vi "Autonomous Independent.vi"() -> ()   [LabVIEW 2020]
doc: "This VI is called when autonomous begins, and will automatically be terminated when autonomous ends. You can carry out timed or sensor driven robot movement independently without needing to return to the caller."
uses:
  <vilib>/Rock Robotics/WPI/ThirdParty/Phoenix-LabVIEW/Motor Controller/Controls/CTRE_Phoenix_MotorControl_ControlMode.ctl
  <vilib>/Rock Robotics/WPI/Solenoid/WPI_SolenoidSetEnum.vi
  <vilib>/Rock Robotics/WPI/Solenoid/WPI_SolenoidValue.ctl
  <vilib>/Rock Robotics/Network Tables/NT Read Number.vi
  <vilib>/Rock Robotics/Network Tables/NT Read String.vi
  <vilib>/Rock Robotics/Network Tables/NT Write Numeric Array.vi
  AutonBoolean.vi
panel:
  out "Ty 24":dbl
  out "Ty 23":dbl
  out "Ty 22":dbl
  out "Ty 21":dbl
  out "Ty 20":dbl
  out "Ty 19":dbl
  out "Ty 18":dbl
  out "Ty 17":dbl
  out "Orange Limit Pressed 10":bool
  out "Blue Limit Pressed 10":bool
  out "Ty 16":dbl
  out "Orange Limit Pressed 9":bool
  out "Blue Limit Pressed 9":bool
  out "Ty 15":dbl
  out "Intake 5":bool
  out "Elevate 5":bool
  out "Ty 14":dbl
  out "Ty 13":dbl
  out "Ty 12":dbl
  out "Ty 11":dbl
  out "Ty 10":dbl
  out "Ty 9":dbl
  out "Orange Limit Pressed 4":bool
  out "Blue Limit Pressed 4":bool
  out "Ty 4":dbl
  out "Orange Limit Pressed 3":bool
  out "Blue Limit Pressed 3":bool
  out "Ty 3":dbl
  out "Intake 2":bool
  out "Elevate 2":bool
  out "Intake":bool
  out "Elevate":bool
  out "Orange Limit Pressed":bool
  out "Blue Limit Pressed":bool
  out "Ty":dbl
  out "Orange Limit Pressed 2":bool
  out "Blue Limit Pressed 2":bool
  out "Ty 2":dbl
  out "Intake 3":bool
  out "Elevate 3":bool
  out "Orange Limit Pressed 5":bool
  out "Blue Limit Pressed 5":bool
  out "Ty 5":dbl
  out "Orange Limit Pressed 6":bool
  out "Blue Limit Pressed 6":bool
  out "Ty 6":dbl
  out "Intake 4":bool
  out "Elevate 4":bool
  out "Orange Limit Pressed 7":bool
  out "Blue Limit Pressed 7":bool
  out "Ty 7":dbl
  out "Orange Limit Pressed 8":bool
  out "Blue Limit Pressed 8":bool
  out "Ty 8":dbl
  # "Be sure to right-click and choose Data Operations>>Make Current Value default if you want to save the array values with the VI"
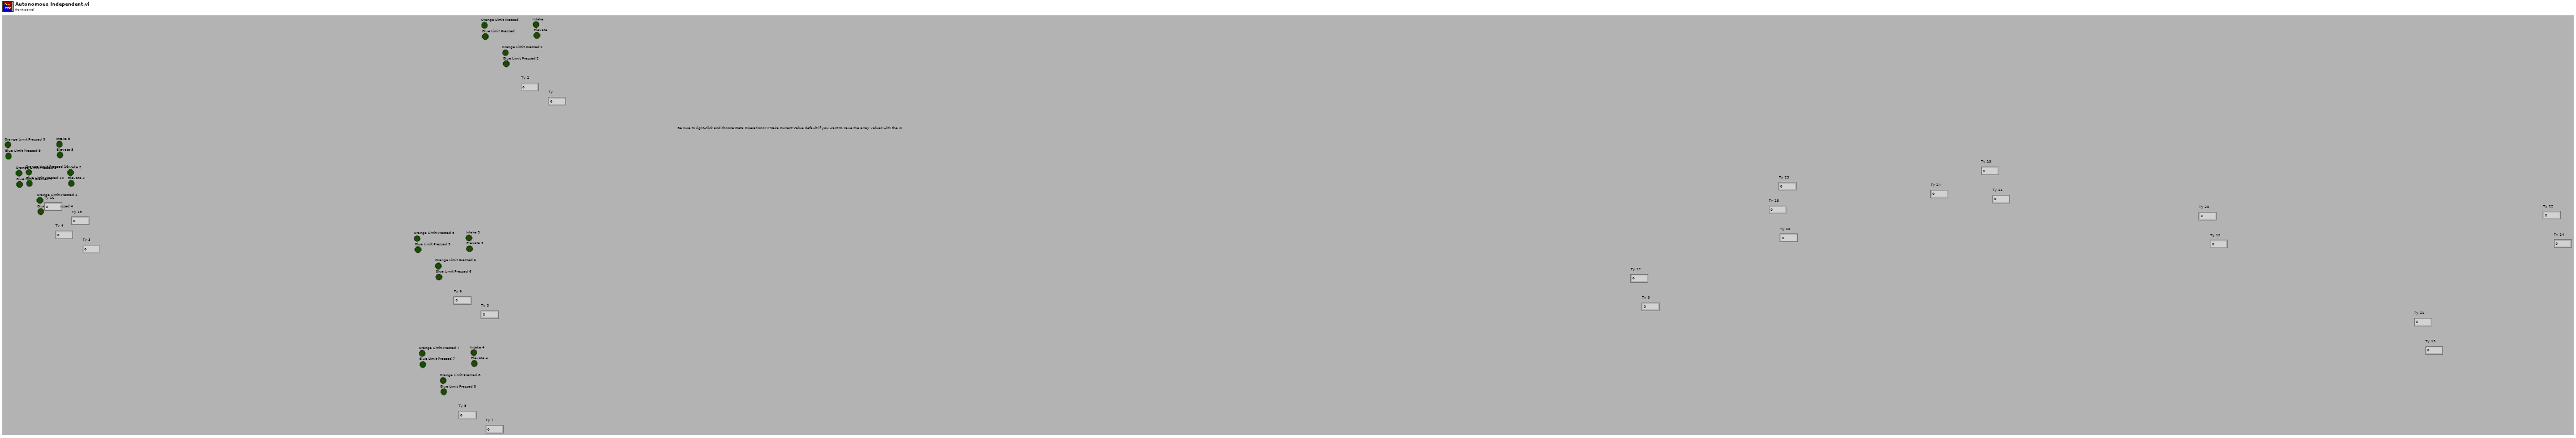
[diagram p1: front panel]
types:
  T1 = typedef "WPI_JoystickDevRef.ctl" = cluster{"Device":T2}
  T2 = typedef "WPI_JoystickDeviceEnum.ctl" = enum16{"USB 0", "USB 1", "USB 2", "USB 3", "USB 4", "USB 5"}
  T3 = typedef "WPI_SolenoidValue.ctl" = enum16{"Off", "On", "Forward", "Reverse"}
  T4 = typedef "WPI_SwitchDevRef.ctl" = cluster{"DevStatus":errorcluster, "DIO Channel":T5, "CntIndex":T6, "Normally Closed":bool}
  T5 = typedef "FPGA_DIOChannel.ctl" = enum8{"DIO 0", "DIO 1", "DIO 2", "DIO 3", "DIO 4", "DIO 5", "DIO 6", "DIO 7", "DIO 8", "DIO 9", "DIO MXP 0", "DIO MXP 1", "DIO MXP 2", "DIO MXP 3", "DIO MXP 4", "DIO MXP 5", "DIO MXP 6", "DIO MXP 7", "DIO MXP 8", "DIO MXP 9", "DIO MXP 10", "DIO MXP 11", "DIO MXP 12", "DIO MXP 13", "DIO MXP 14", "DIO MXP 15", "SPI Port CS1", "SPI Port CS2", "SPI Port CS3", "SPI Port MISO", "SPI Port MOSI", "Invalid"}
  T6 = typedef "FPGA_CounterCtrSystemIndex.ctl" = enum8{"Ctr 0", "Ctr 1", "Ctr 2", "Ctr 3", "Ctr 4", "Ctr 5", "Ctr 6", "Ctr 7", "Invalid"}
  T7 = typedef "WPI_SolenoidDevRef.ctl" = cluster{"DevStatus":errorcluster, "Pneumatics Control Module":u8, "Forward Solenoid Channel":T8, "Reverse Solenoid Channel":T8}
  T8 = typedef "WPI_SolenoidChannel.ctl" = enum8{"Solenoid 0", "Solenoid 1", "Solenoid 2", "Solenoid 3", "Solenoid 4", "Solenoid 5", "Solenoid 6", "Solenoid 7", "Solenoid 8", "Solenoid 9", "Solenoid 10", "Solenoid 11", "Solenoid 12", "Solenoid 13", "Solenoid 14", "Solenoid 15", "Invalid"}
  T9 = typedef "WPI_MotorControlDeviceRef.ctl" = cluster{"DeviceStatus":errorcluster, "Type":T10, "PWM":cluster{"PWM Channel":T11, "DeadBand":T12}, "CAN":cluster{"Device Number":u8, "SetOutput VI Ref":variant, "GetOutput VI Ref":variant, "Enable VI Ref":variant, "Disable VI Ref":variant, "Data":variant}, "Invert":bool, "DIO PWM":cluster{"PWM \"Enable\" Channel":T11, "DIOChannel":T5, "PWM Rate":dbl}}
  T10 = typedef "WPI_MotorControlType.ctl" = enum16{"PWM", "CAN", "DIO PWM"}
  T11 = typedef "FPGA_DIOPWMChannel.ctl" = enum8{"PWM 0", "PWM 1", "PWM 2", "PWM 3", "PWM 4", "PWM 5", "PWM 6", "PWM 7", "PWM 8", "PWM 9", "PWM MXP 0", "PWM MXP 1", "PWM MXP 2", "PWM MXP 3", "PWM MXP 4", "PWM MXP 5", "PWM MXP 6", "PWM MXP 7", "PWM MXP 8", "PWM MXP 9", "Invalid"}
  T12 = typedef "WPI_PWMDeadband.ctl" = cluster{"Name":string, "maxPositivePwm":i32, "minPositivePwm":i32, "centerPwm":i32, "maxNegativePwm":i32, "minNegativePwm":i32, "angularRange":u16}
  T13 = typedef "CTRE_Phoenix_MotorControl_ControlMode.ctl" = u16
  T14 = typedef "Trajectory Data.ctl" = cluster{"Segment Name":string, "Type":T15, "Traj Pos Points":cluster{"x":dbl, "y":dbl, "th":dbl}[], "Traj Vel Points":cluster{"V":dbl, "Omega":dbl, "V vector":cluster{"y":dbl, "x":dbl}}[], "Accel Index":i32, "Decel Index":i32}[]
  T15 = typedef "Segment Type.ctl" = enum16{"Accel Straight", "Const Straight", "Blend", "Circle", "Bezier"}
  T16 = typedef "Overrides.ctl" = cluster{"Count":string, "Angular Override":dbl, "Enabled?":bool, "Velocity Override":dbl, "Angle Override":dbl}[]
  T17 = typedef "Angluar Limits.ctl" = cluster{"Velocity (deg/s)":dbl, "Accel (deg/s^2)":dbl, "Jerk (deg/s^3)":dbl}
  T18 = cluster{"Sample Period (s)":dbl, cluster{"Velocity (fps)":dbl, "Accel (fps^2)":dbl, "Jerk (fps^3)":dbl, "StoopidFast (fps)":dbl}, "Conditions":cluster{"vInitial (fps)":dbl, "vFinal (fps)":dbl}, "Overrides":T16, "Angular Limits":T17}
  T19 = cluster{"Velocity (fps)":dbl, "Accel (fps^2)":dbl, "Jerk (fps^3)":dbl, "StoopidFast (fps)":dbl}
  T20 = cluster{"V":dbl, "Omega":dbl, "V vector":cluster{"y":dbl, "x":dbl}}[]
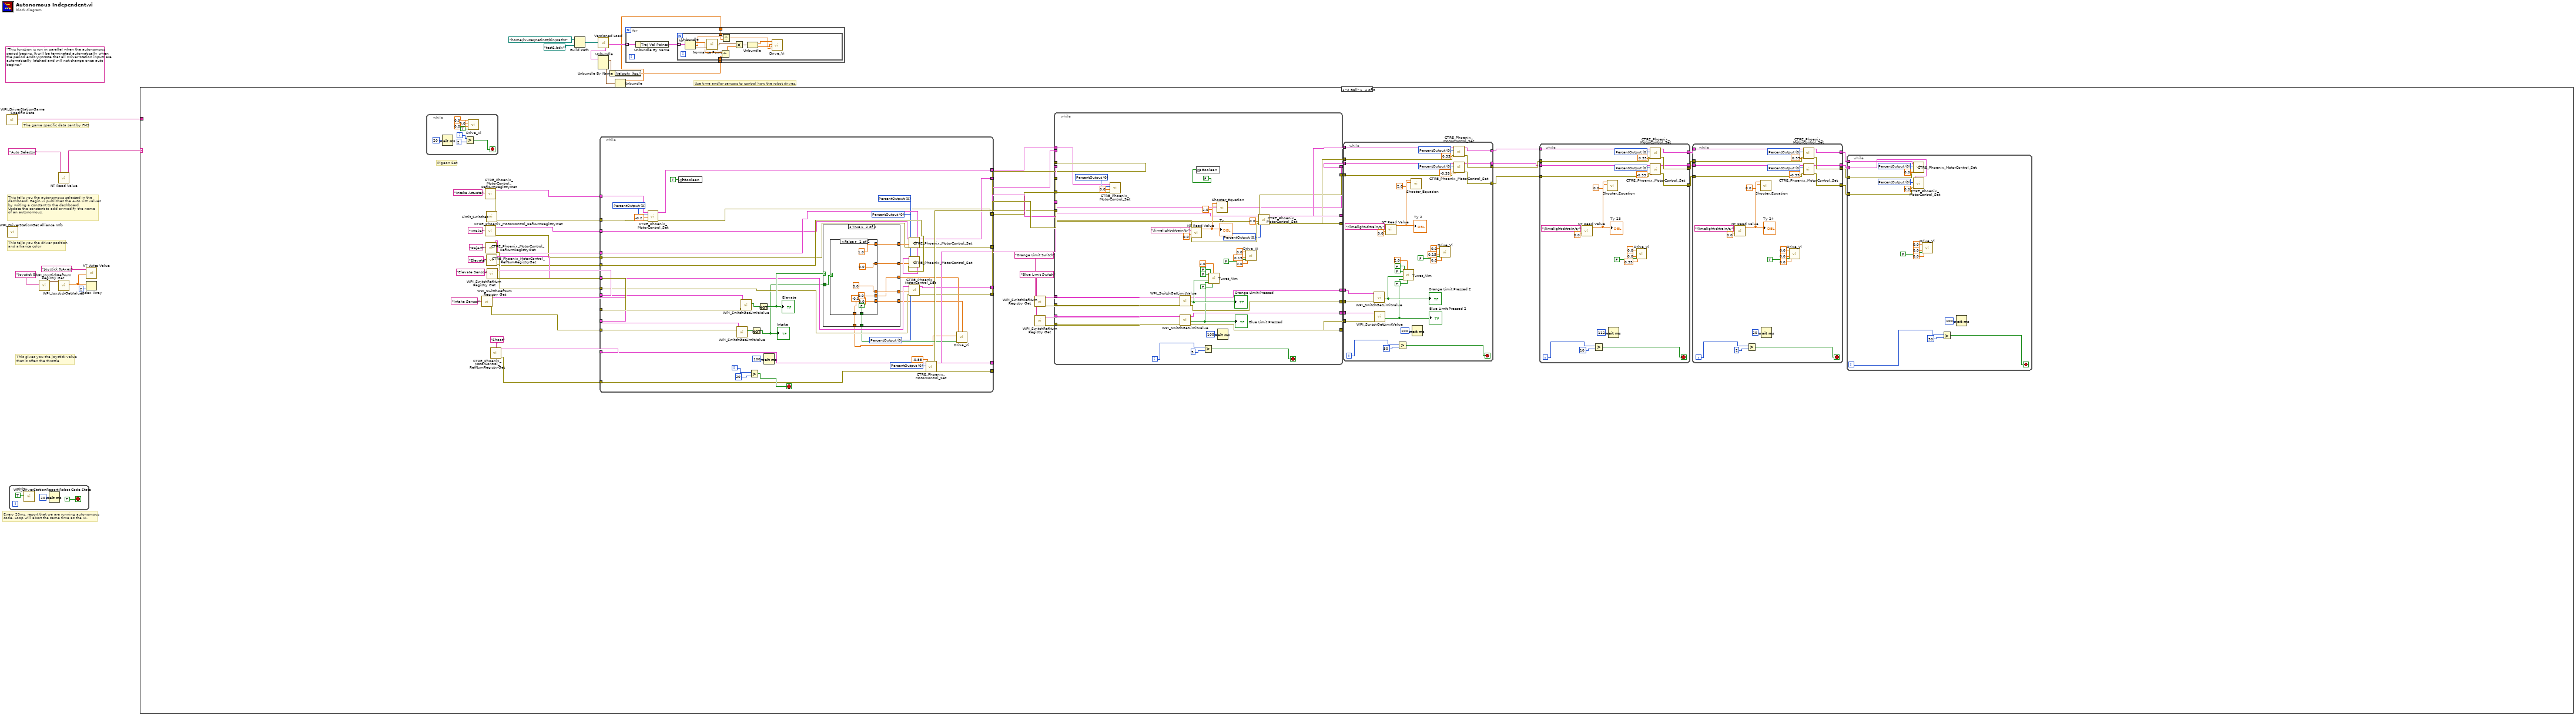
[diagram p0: block diagram]
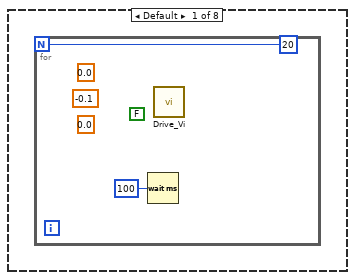
[diagram p2: hidden frame]
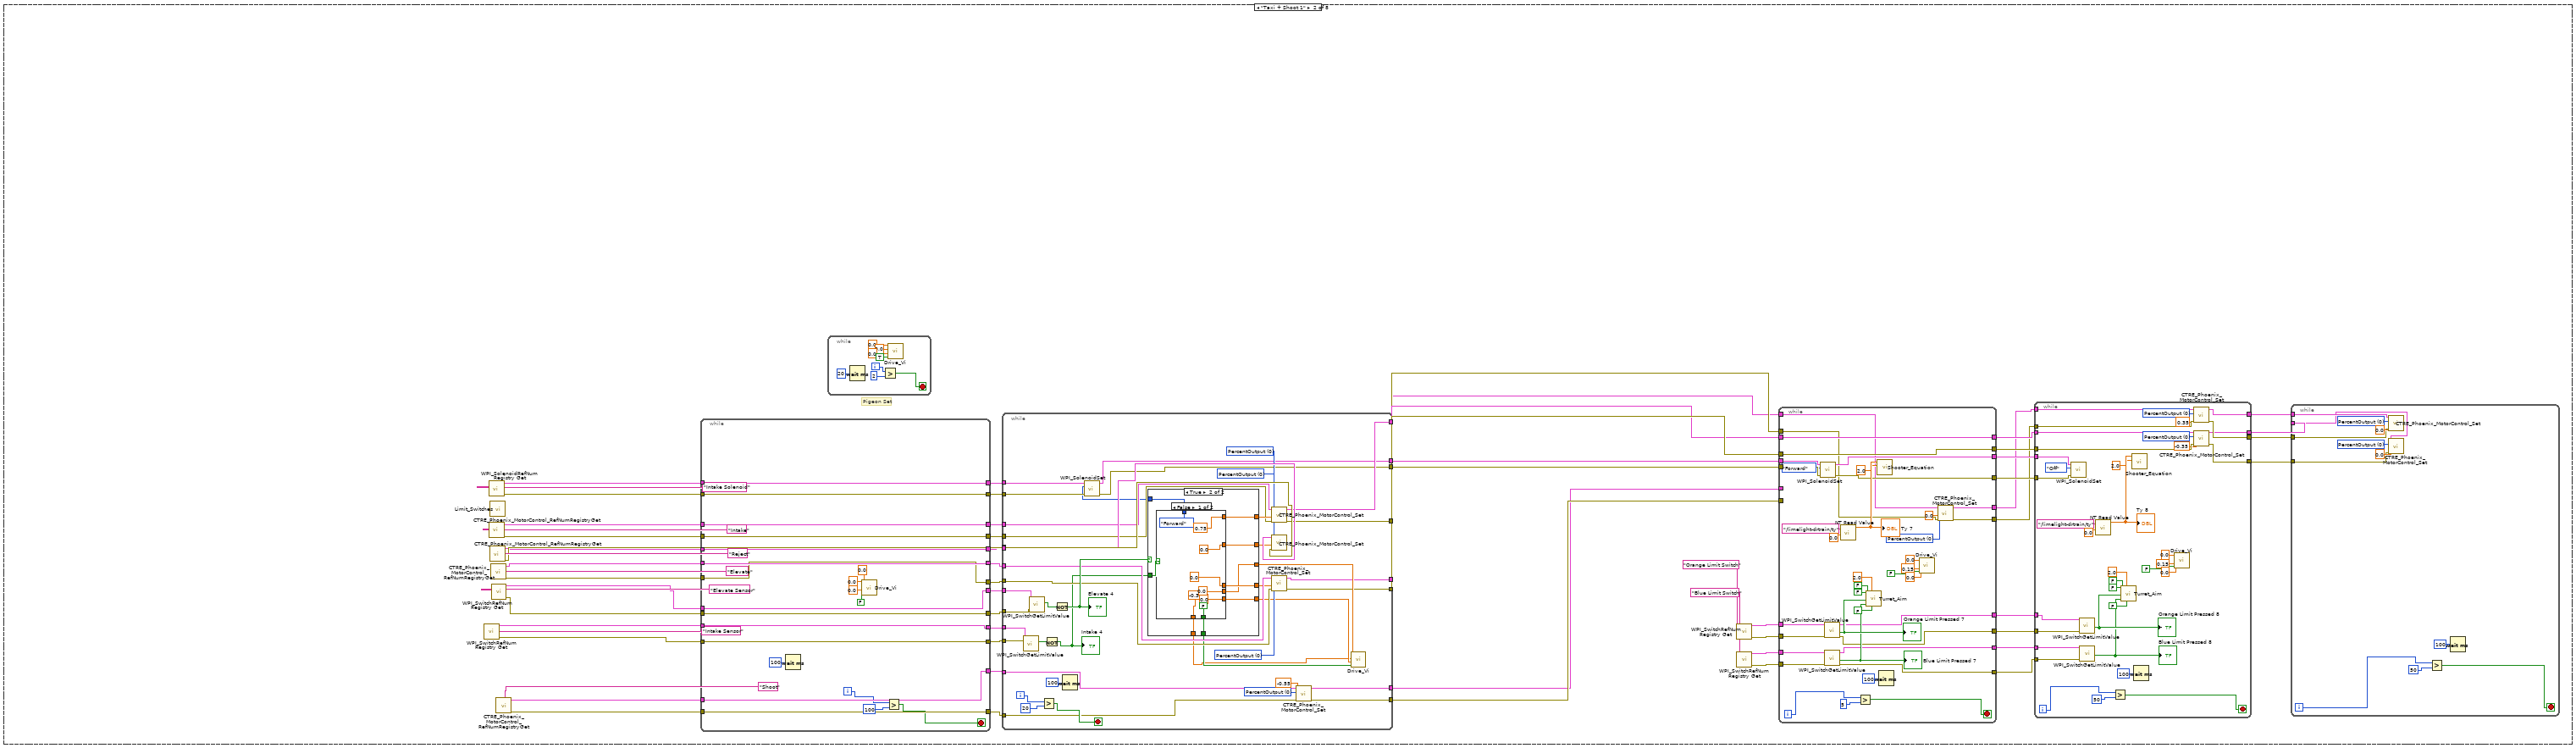
[diagram p3: hidden frame]
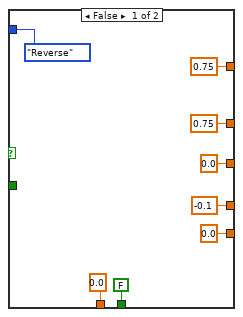
[diagram p4: hidden frame]
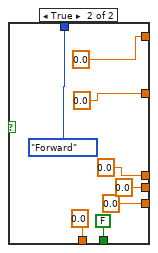
[diagram p5: hidden frame]
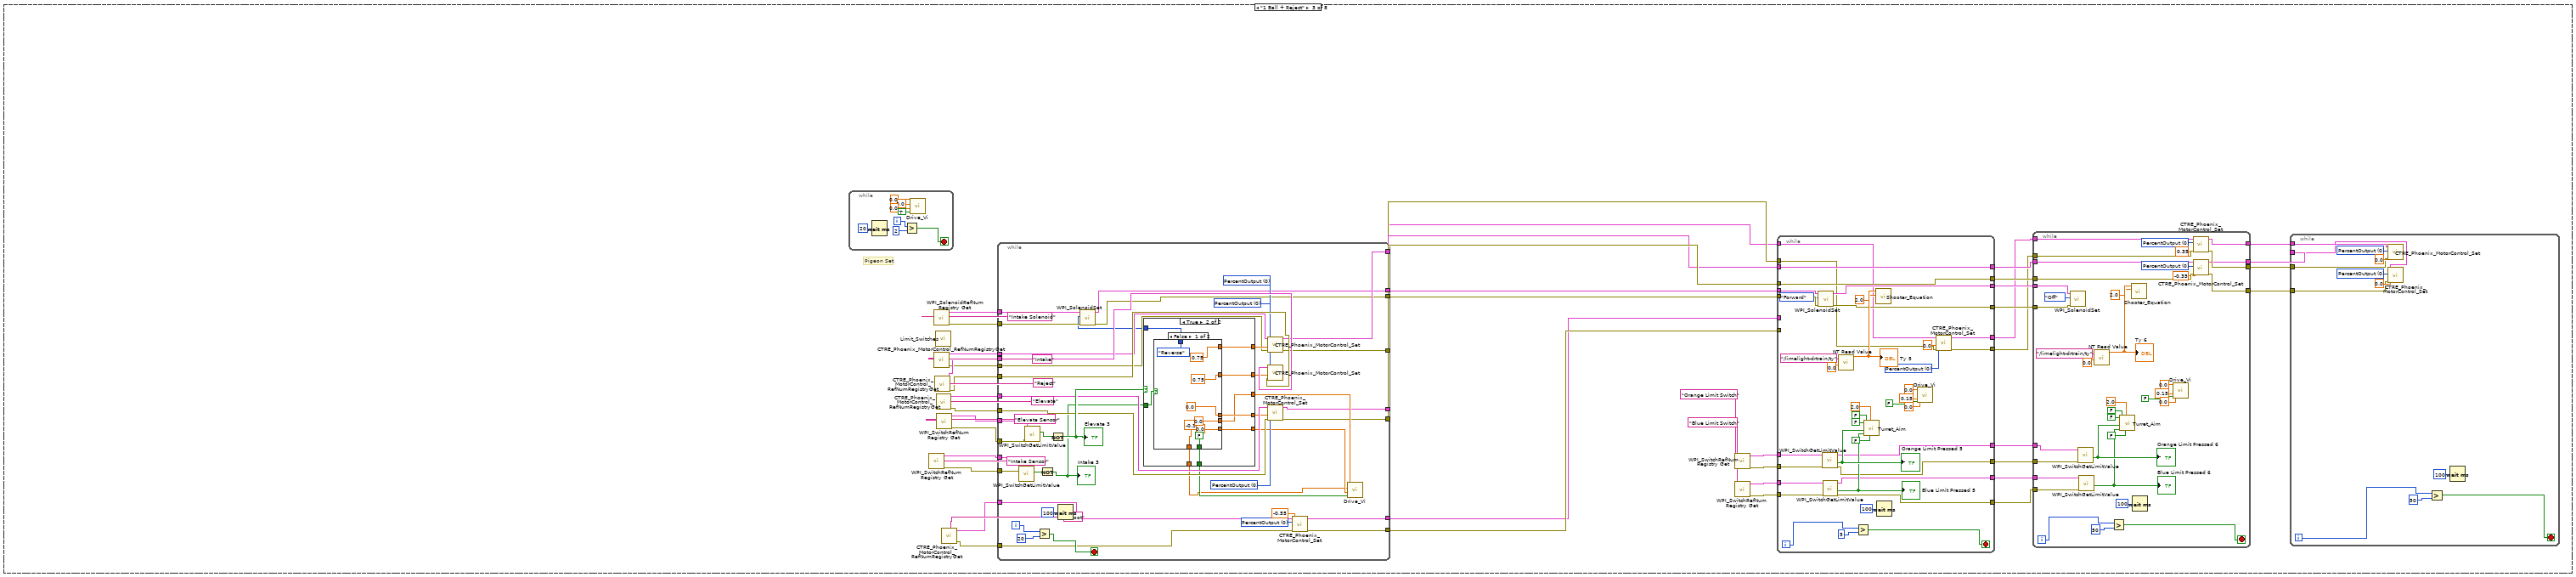
[diagram p6: hidden frame]
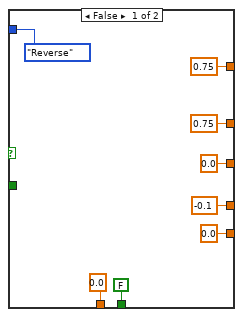
[diagram p7: hidden frame]
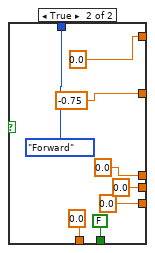
[diagram p8: hidden frame]
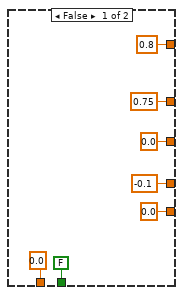
[diagram p9: hidden frame]
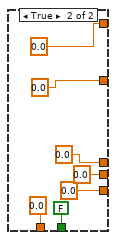
[diagram p10: hidden frame]
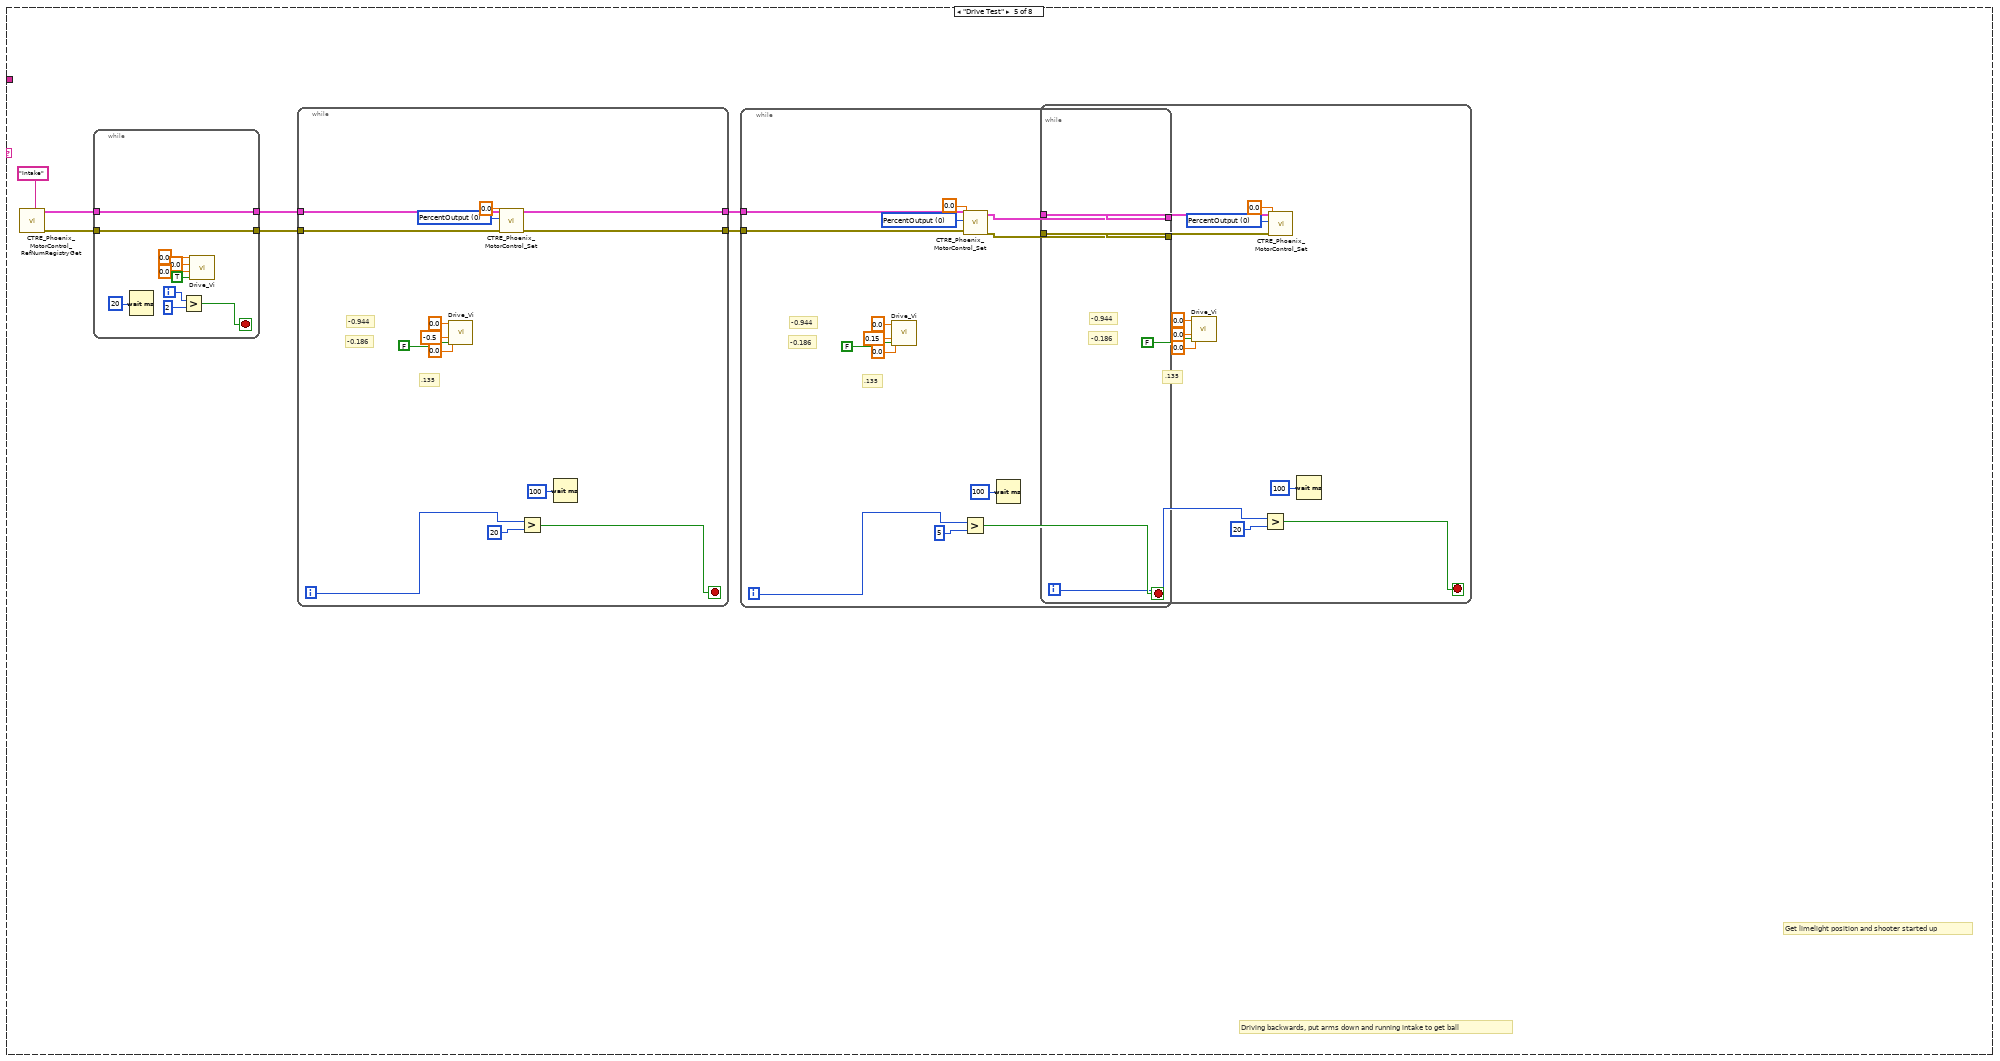
[diagram p11: hidden frame]
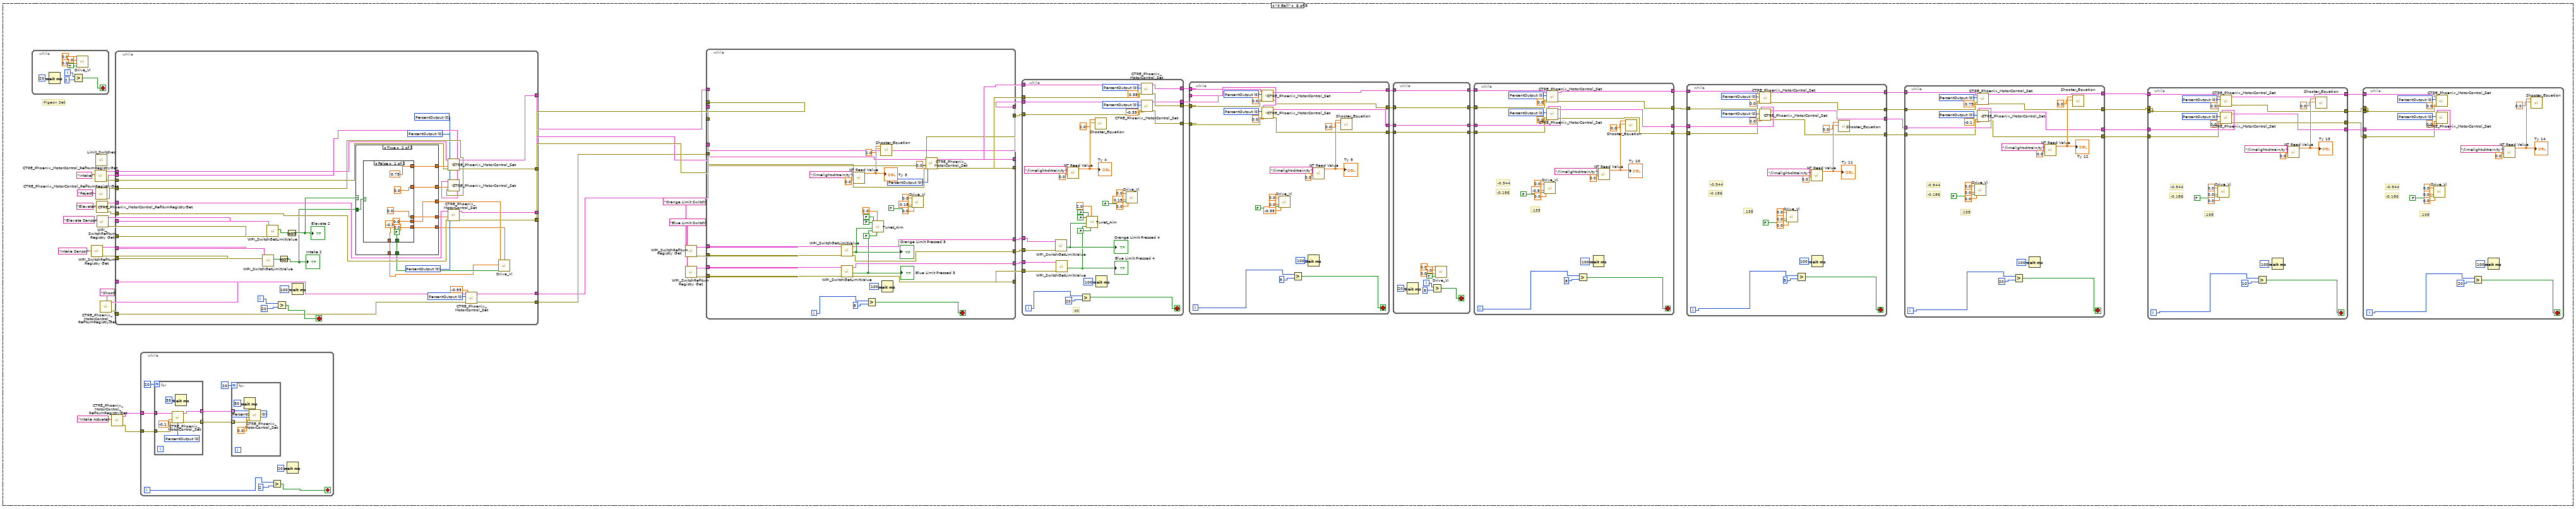
[diagram p12: hidden frame]
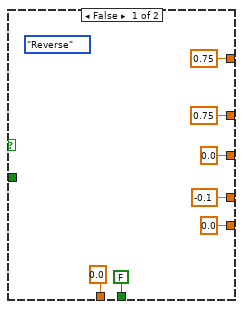
[diagram p13: hidden frame]
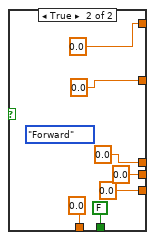
[diagram p14: hidden frame]
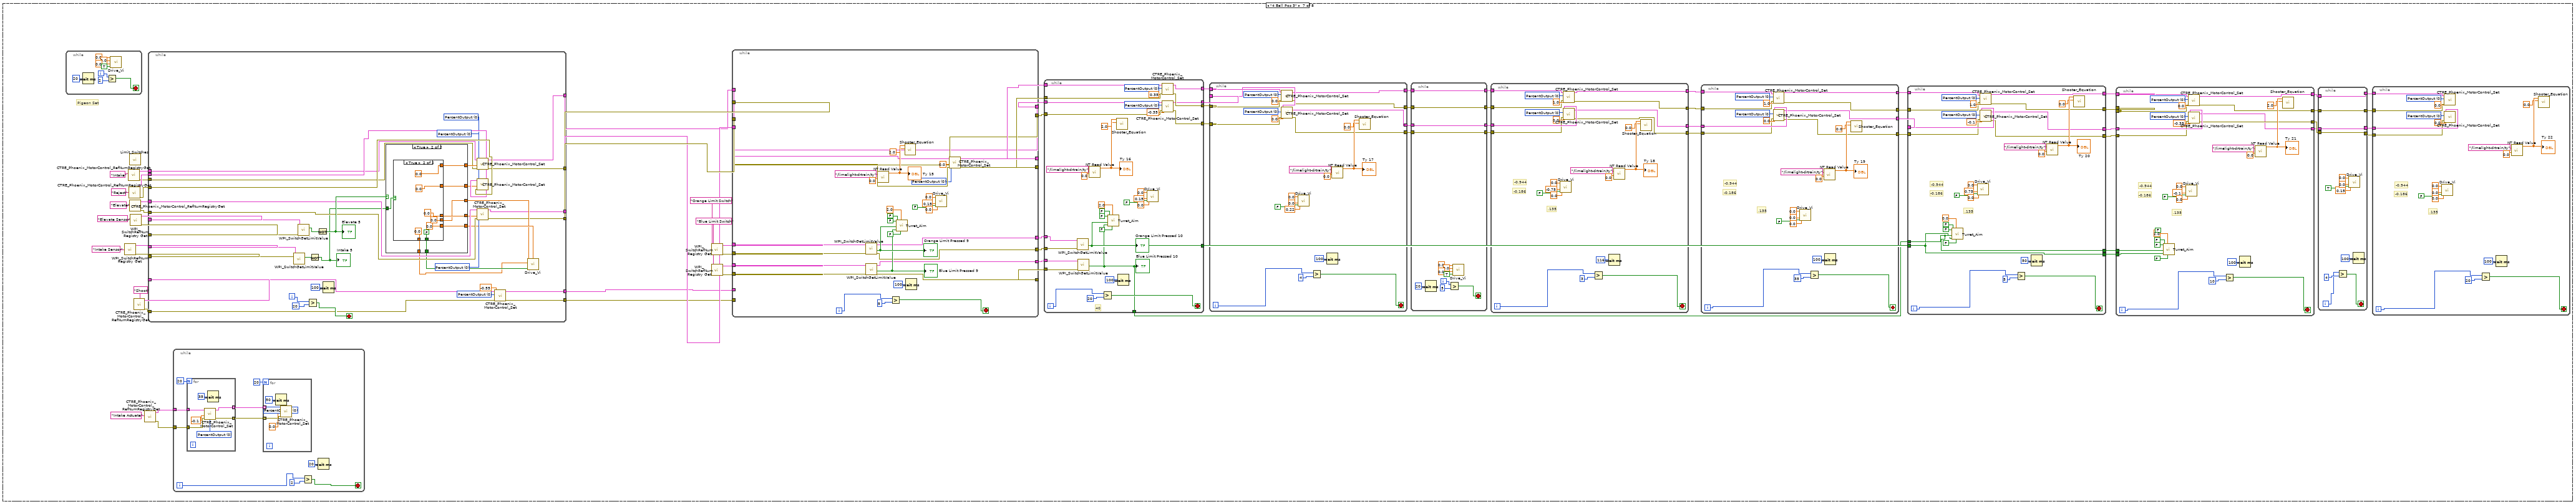
[diagram p15: hidden frame]
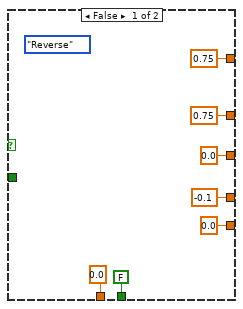
[diagram p16: hidden frame]
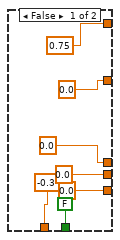
[diagram p17: hidden frame]
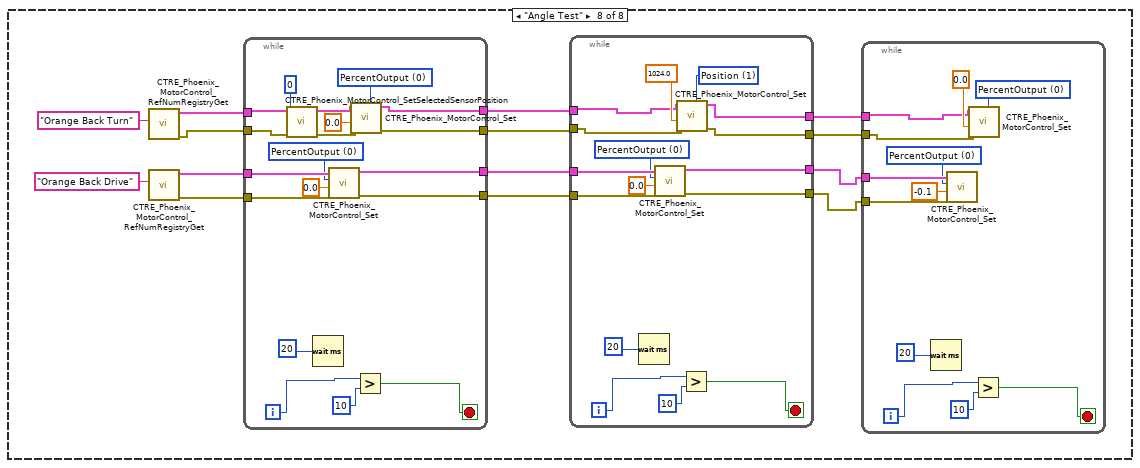
[diagram p18: hidden frame]
diagram:
  (unwired) "This function is run in parallel when the autonomous period begins. It will be terminated automatically when the period ends.\n\nNote that all Driver Station inputs are automatically latched and will not change once auto begins."
  # "The game specific data sent by FMS"
  # "This tells you the autonomous selected in the \ndashboard. Begin.vi publishes the Auto List values\nby writing a constant to the dashboard.\nUpdate the constant to add or modify the name\nof an autonomous."
  # "Every 20ms, report that we are running autonomous\ncode. Loop will abort the same time as the VI."
  # "This gives you the joystick value\nthat is often the throttle"
  # "Use time and/or sensors to control how the robot drives."
  # "This tells you the driver position\nand alliance color"
  n1 = call <vilib>:"WPI_DriverStationGame Specific Data.vi"() -> ("Game Specific Data"=w10:string)  [unwired: 11 in]
  n2 = call <vilib>:"WPI_DriverStationGet Alliance Info.vi"() -> ()  [unwired: 12 out]
  n3 = while {
    stop <- FALSE stop-if-true
    n4 = call <vilib>:"WPI_DriverStationReport Robot Code State.vi"("Autonomous"=TRUE) -> ()  [unwired: 10 in, 1 out]
    n5 = Wait (ms)(milliseconds to wait=u32 20) -> ()  [unwired: 1 out]
  }
  n6 = call <vilib>:"WPI_JoystickRefNum Registry Get.vi"("refnum name"="Joystick 0") -> ("JoystickDevRef"=w16:T1)  [unwired: 1 in, 9 out]
  n7 = call <vilib>:"WPI_JoystickGetValues.vi"("JoystickDevRef"=w16) -> ("Axes"=w12:dbl[])  [unwired: 6 in, 4 out]
  n8 = call-poly <vilib>:"NT Read Value.vi"("Name"="Auto Selector") -> ("String"=w13:string)  [unwired: 9 in, 1 out]
  n9 = call-poly <vilib>:"NT Write Value.vi"("Numeric Array"=w12, "Name"="Joystick 0/Axes") -> ()  [unwired: 9 in, 1 out]
  n10 = Index Array(array=w12, index=2) -> ()  [unwired: 1 out]
  n11 = case shown="\"2 Ball\"" w13 {
    tunnel: w10 -> [_ _ _ _ _ _ _ _]
    frame Default {
      n12 = for {
        N: 20 -> [_]
        (unwired) FALSE ("Middle Thumb")
        (unwired) 0.0 ("Z")
        (unwired) -0.1 ("Y")
        (unwired) 0.0 ("X")
        n13 = Wait (ms)(milliseconds to wait=u32 100) -> ()  [unwired: 1 out]
        n14 = call "Drive_Vi.vi"() -> ()  [unwired: 12 in]
      }
    }
    frame "Taxi + Shoot 1" {
      # "Pigeon Set"
      n15 = call <vilib>:"WPI_SwitchRefNum Registry Get.vi"("refnum name"="Intake Sensor") -> ("error out"=w27:errorcluster, "SwitchDevRef"=w29:T4)  [unwired: 9 in]
      n16 = call <vilib>:"WPI_SolenoidRefNum Registry Get.vi"("refnum name"="Intake Solenoid") -> ("error out"=w46:errorcluster, "SolenoidDevRef"=w48:T7)  [unwired: 9 in]
      n17 = call <vilib>:"CTRE_Phoenix_MotorControl_RefNumRegistryGet.vi"("refnum name"="Intake") -> ("error out"=w41:errorcluster, "PhoenixMotorControlDevRef"=w43:T9)  [unwired: 9 in]
      n18 = call <vilib>:"CTRE_Phoenix_MotorControl_RefNumRegistryGet.vi"("refnum name"="Reject") -> ("error out"=w77:errorcluster, "PhoenixMotorControlDevRef"=w39:T9)  [unwired: 9 in]
      n19 = call "Limit_Switches.vi"() -> ()  [unwired: 10 in, 2 out]
      n20 = call <vilib>:"CTRE_Phoenix_MotorControl_RefNumRegistryGet.vi"("refnum name"="Elevate") -> ("error out"=w35:errorcluster, "PhoenixMotorControlDevRef"=w37:T9)  [unwired: 9 in]
      n21 = call <vilib>:"WPI_SwitchRefNum Registry Get.vi"("refnum name"="Elevate Sensor") -> ("error out"=w31:errorcluster, "SwitchDevRef"=w33:T4)  [unwired: 9 in]
      n22 = call <vilib>:"CTRE_Phoenix_MotorControl_RefNumRegistryGet.vi"("refnum name"="Shoot") -> ("error out"=w23:errorcluster, "PhoenixMotorControlDevRef"=w26:T9)  [unwired: 9 in]
      n23 = while {
        tunnel: [w101] -> w47
        tunnel: w48 -> [w101]
        tunnel: [w100] -> w45
        tunnel: w46 -> [w100]
        tunnel: [w99] -> w44
        tunnel: w43 -> [w99]
        tunnel: [w98] -> w42
        tunnel: w41 -> [w98]
        tunnel: [w97] -> w40
        tunnel: w39 -> [w97]
        tunnel: [w96] -> w38
        tunnel: w37 -> [w96]
        tunnel: [w95] -> w36
        tunnel: w35 -> [w95]
        tunnel: [w94] -> w34
        tunnel: w33 -> [w94]
        tunnel: [w93] -> w32
        tunnel: w31 -> [w93]
        tunnel: [w92] -> w30
        tunnel: w29 -> [w92]
        tunnel: [w91] -> w28
        tunnel: w27 -> [w91]
        tunnel: [w90] -> w25
        tunnel: w26 -> [w90]
        tunnel: [w89] -> w24
        tunnel: w23 -> [w89]
        i -> [w85]
        stop <- w87 stop-if-true
        n24 = Wait (ms)(milliseconds to wait=u32 100) -> ()  [unwired: 1 out]
        n25 = call "Drive_Vi.vi"("Middle Thumb"=FALSE, "Z"=0.0, "Y"=0.0, "X"=0.0) -> ()  [unwired: 8 in]
        n26 = Greater?(x=w85, y=100) -> (0:w87:bool)
      }
      n27 = while {
        i -> [w275]
        stop <- w276 stop-if-true
        n28 = Wait (ms)(milliseconds to wait=u32 20) -> ()  [unwired: 1 out]
        n29 = Greater?(x=w275, y=2) -> (0:w276:bool)
        n30 = call "Drive_Vi.vi"("Middle Thumb"=TRUE, "Z"=0.0, "Y"=0.0, "X"=0.0) -> ()  [unwired: 8 in]
      }
      n31 = while {
        tunnel: w32 -> [w230]
        tunnel: w34 -> [w229]
        tunnel: w28 -> [w228]
        tunnel: w30 -> [w227]
        tunnel: w45 -> [w226]
        tunnel: w47 -> [w225]
        tunnel: w36 -> [w222]
        tunnel: w38 -> [w221]
        tunnel: w77 -> [w220]
        tunnel: w40 -> [w219]
        tunnel: w42 -> [w218]
        tunnel: w44 -> [w217]
        tunnel: [w205] -> w70
        tunnel: [w204] -> w69
        tunnel: [w203] -> w68
        tunnel: [w202] -> w67
        tunnel: w24 -> [w201]
        tunnel: w25 -> [w200]
        tunnel: [w197] -> w66
        tunnel: [w196] -> w65
        tunnel: [w195] -> w58
        tunnel: [w194] -> w57
        i -> [w233]
        stop <- w234 stop-if-true
        w199 = T13 0 items=["PercentOutput"=0, "Position"=1, "Velocity"=2, "Current"=3, "Follower"=5, "MotionProfile"=6, "MotionMagic"=7, "MotionProfileArc"=10, "Disabled"=15] ("Control Mode")
        w211 = T13 0 items=["PercentOutput"=0, "Position"=1, "Velocity"=2, "Current"=3, "Follower"=5, "MotionProfile"=6, "MotionMagic"=7, "MotionProfileArc"=10, "Disabled"=15] ("Control Mode")
        w212 = T13 0 items=["PercentOutput"=0, "Position"=1, "Velocity"=2, "Current"=3, "Follower"=5, "MotionProfile"=6, "MotionMagic"=7, "MotionProfileArc"=10, "Disabled"=15] ("Control Mode")
        w213 = T13 0 items=["PercentOutput"=0, "Position"=1, "Velocity"=2, "Current"=3, "Follower"=5, "MotionProfile"=6, "MotionMagic"=7, "MotionProfileArc"=10, "Disabled"=15] ("Control Mode")
        n32 = call <vilib>:"WPI_SwitchGetLimitValue.vi"("error in (no error)"=w228, "SwitchDevRef"=w227) -> ("Switch Pressed"=w231:bool)  [unwired: 7 in, 2 out]
        n33 = call <vilib>:"WPI_SwitchGetLimitValue.vi"("error in (no error)"=w230, "SwitchDevRef"=w229) -> ("Switch Pressed"=w232:bool)  [unwired: 7 in, 2 out]
        n34 = Greater?(x=w233, y=20) -> (0:w234:bool)
        n35 = Not(x=w231) -> (.not. x?=w216:bool)
        "Intake 4" <- w216
        n36 = Not(x=w232) -> (.not. x?=w224:bool)
        "Elevate 4" <- w224
        n37 = Wait (ms)(milliseconds to wait=u32 100) -> ()  [unwired: 1 out]
        n38 = case shown="True" w224 {
          tunnel: [0.75 ("Output") w253] -> w223
          tunnel: w216 -> [_ w250]
          tunnel: [0.75 ("Output") w252] -> w215
          tunnel: [-0.1 ("Output") w251] -> w214
          tunnel: [FALSE ("Middle Thumb") w249] -> w210
          tunnel: [0.0 ("Z") w248] -> w209
          tunnel: [0.0 ("Y") w247] -> w208
          tunnel: [0.0 ("X") w246] -> w207
          tunnel: [WPI_SolenoidValue."Reverse" ("Value") w245] -> w206
          frame False {
          }
          frame True {
            n39 = case shown="False" w250 {
              tunnel: [0.75 ("Output") 0.0 ("Output")] -> w253
              tunnel: [0.0 ("Output") 0.0 ("Output")] -> w252
              tunnel: [0.0 ("Output") 0.0 ("Output")] -> w251
              tunnel: [FALSE ("Middle Thumb") FALSE ("Middle Thumb")] -> w249
              tunnel: [0.0 ("Z") 0.0 ("Z")] -> w248
              tunnel: [-0.3 ("Y") 0.0 ("Y")] -> w247
              tunnel: [0.0 ("X") 0.0 ("X")] -> w246
              tunnel: [WPI_SolenoidValue."Forward" ("Value") WPI_SolenoidValue."Forward" ("Value")] -> w245
              frame False {
              }
              frame True {
              }
            }
          }
        }
        n40 = call-poly <vilib>:"WPI_SolenoidSet.vi"("error in (no error)"=w226, "Value"=w206, "SolenoidDevRef"=w225) -> ("error out"=w194:errorcluster, "SolenoidDevRef"=w195:T7)  [unwired: 7 in]
        n41 = call <vilib>:"CTRE_Phoenix_MotorControl_Set.vi"("error in (no error)"=w218, "Output"=w223, "Control Mode"=w211, "PhoenixMotorControlDevRef"=w217) -> ("error out"=w203:errorcluster, "PhoenixMotorControlDevRef"=w202:T9)  [unwired: 6 in]
        n42 = call <vilib>:"CTRE_Phoenix_MotorControl_Set.vi"("error in (no error)"=w220, "Output"=w215, "Control Mode"=w212, "PhoenixMotorControlDevRef"=w219) -> ()  [unwired: 6 in, 2 out]
        n43 = call <vilib>:"CTRE_Phoenix_MotorControl_Set.vi"("error in (no error)"=w222, "Output"=w214, "Control Mode"=w213, "PhoenixMotorControlDevRef"=w221) -> ("error out"=w205:errorcluster, "PhoenixMotorControlDevRef"=w204:T9)  [unwired: 6 in]
        n44 = call <vilib>:"CTRE_Phoenix_MotorControl_Set.vi"("error in (no error)"=w201, "Output"=-0.55, "Control Mode"=w199, "PhoenixMotorControlDevRef"=w200) -> ("error out"=w197:errorcluster, "PhoenixMotorControlDevRef"=w196:T9)  [unwired: 6 in]
        n45 = call "Drive_Vi.vi"("Middle Thumb"=w210, "Z"=w209, "Y"=w208, "X"=w207) -> ()  [unwired: 8 in]
      }
      n46 = call <vilib>:"WPI_SwitchRefNum Registry Get.vi"("refnum name"="Orange Limit Switch") -> ("error out"=w72:errorcluster, "SwitchDevRef"=w71:T4)  [unwired: 9 in]
      n47 = call <vilib>:"WPI_SwitchRefNum Registry Get.vi"("refnum name"="Blue Limit Switch") -> ("error out"=w74:errorcluster, "SwitchDevRef"=w73:T4)  [unwired: 9 in]
      n48 = while {
        tunnel: w66 -> [_]
        tunnel: w65 -> [_]
        tunnel: w74 -> [w191]
        tunnel: w73 -> [w190]
        tunnel: w72 -> [w189]
        tunnel: w71 -> [w188]
        tunnel: w70 -> [w167]
        tunnel: w69 -> [w166]
        tunnel: w68 -> [w157]
        tunnel: w67 -> [w158]
        tunnel: [w171] -> w64
        tunnel: [w170] -> w63
        tunnel: [w169] -> w62
        tunnel: [w168] -> w61
        tunnel: [w167] -> w60
        tunnel: [w166] -> w59
        tunnel: w58 -> [w165]
        tunnel: w57 -> [w164]
        tunnel: [w162] -> w56
        tunnel: [w161] -> w55
        tunnel: [w160] -> w54
        tunnel: [w159] -> w53
        i -> [w177]
        stop <- w176 stop-if-true
        w156 = T13 0 items=["PercentOutput"=0, "Position"=1, "Velocity"=2, "Current"=3, "Follower"=5, "MotionProfile"=6, "MotionMagic"=7, "MotionProfileArc"=10, "Disabled"=15] ("Control Mode")
        n49 = call-poly <vilib>:"WPI_SolenoidSet.vi"("error in (no error)"=w164, "Value"=WPI_SolenoidValue."Forward", "SolenoidDevRef"=w165) -> ("error out"=w161:errorcluster, "SolenoidDevRef"=w162:T7)  [unwired: 7 in]
        n50 = call <vilib>:"WPI_SwitchGetLimitValue.vi"("error in (no error)"=w189, "SwitchDevRef"=w188) -> ("error out"=w168:errorcluster, "Switch Pressed"=w187:bool, "SwitchDevRef"=w169:T4)  [unwired: 7 in]
        "Orange Limit Pressed 7" <- w187
        n51 = call <vilib>:"WPI_SwitchGetLimitValue.vi"("error in (no error)"=w191, "SwitchDevRef"=w190) -> ("error out"=w170:errorcluster, "Switch Pressed"=w186:bool, "SwitchDevRef"=w171:T4)  [unwired: 7 in]
        "Blue Limit Pressed 7" <- w186
        n52 = call-poly <vilib>:"NT Read Value.vi"("Default Value"=0.0, "Name"="/limelight-drtrain/ty") -> ("Numeric"=w181:dbl)  [unwired: 8 in, 1 out]
        "Ty 7" <- w181
        n53 = Greater?(x=w177, y=5) -> (0:w176:bool)
        n54 = call "Turret_Aim.vi"("View Button"=FALSE ("Driver Right Thumb"), "Left Trigger"=2.0, "Orange Limit Pressed"=w186, "Blue Limit Pressed"=w187, "Right Bumper"=FALSE, "Left Bumper"=FALSE) -> ()  [unwired: 6 in]
        n55 = call "Shooter_Equation.vi"("Right Trigger"=2.0, "Ty"=w181) -> ()  [unwired: 10 in]
        n56 = Wait (ms)(milliseconds to wait=u32 100) -> ()  [unwired: 1 out]
        n57 = call "Drive_Vi.vi"("Middle Thumb"=FALSE, "Z"=0.0, "Y"=0.15, "X"=0.0) -> ()  [unwired: 8 in]
        n58 = call <vilib>:"CTRE_Phoenix_MotorControl_Set.vi"("error in (no error)"=w157, "Output"=0.0, "Control Mode"=w156, "PhoenixMotorControlDevRef"=w158) -> ("error out"=w159:errorcluster, "PhoenixMotorControlDevRef"=w160:T9)  [unwired: 6 in]
      }
      n59 = while {
        tunnel: w63 -> [w152]
        tunnel: w64 -> [w151]
        tunnel: w61 -> [w150]
        tunnel: w60 -> [w137]
        tunnel: w59 -> [w136]
        tunnel: w53 -> [w135]
        tunnel: w54 -> [w134]
        tunnel: w62 -> [w125]
        tunnel: w56 -> [w124]
        tunnel: w55 -> [w123]
        tunnel: [w121] -> w52
        tunnel: [w120] -> w51
        tunnel: [w119] -> w50
        tunnel: [w118] -> w49
        i -> [w139]
        stop <- w138 stop-if-true
        w132 = T13 0 items=["PercentOutput"=0, "Position"=1, "Velocity"=2, "Current"=3, "Follower"=5, "MotionProfile"=6, "MotionMagic"=7, "MotionProfileArc"=10, "Disabled"=15] ("Control Mode")
        w133 = T13 0 items=["PercentOutput"=0, "Position"=1, "Velocity"=2, "Current"=3, "Follower"=5, "MotionProfile"=6, "MotionMagic"=7, "MotionProfileArc"=10, "Disabled"=15] ("Control Mode")
        n60 = call-poly <vilib>:"WPI_SolenoidSet.vi"("error in (no error)"=w123, "Value"=WPI_SolenoidValue."Off", "SolenoidDevRef"=w124) -> ()  [unwired: 7 in, 2 out]
        n61 = call <vilib>:"WPI_SwitchGetLimitValue.vi"("error in (no error)"=w150, "SwitchDevRef"=w125) -> ("Switch Pressed"=w149:bool)  [unwired: 7 in, 2 out]
        "Orange Limit Pressed 8" <- w149
        n62 = call <vilib>:"WPI_SwitchGetLimitValue.vi"("error in (no error)"=w152, "SwitchDevRef"=w151) -> ("Switch Pressed"=w148:bool)  [unwired: 7 in, 2 out]
        "Blue Limit Pressed 8" <- w148
        n63 = call-poly <vilib>:"NT Read Value.vi"("Default Value"=0.0, "Name"="/limelight-drtrain/ty") -> ("Numeric"=w143:dbl)  [unwired: 8 in, 1 out]
        "Ty 8" <- w143
        n64 = Greater?(x=w139, y=50) -> (0:w138:bool)
        n65 = call "Turret_Aim.vi"("View Button"=FALSE ("Driver Right Thumb"), "Left Trigger"=2.0, "Orange Limit Pressed"=w148, "Blue Limit Pressed"=w149, "Right Bumper"=FALSE, "Left Bumper"=FALSE) -> ()  [unwired: 6 in]
        n66 = call "Shooter_Equation.vi"("Right Trigger"=2.0, "Ty"=w143) -> ()  [unwired: 10 in]
        n67 = Wait (ms)(milliseconds to wait=u32 100) -> ()  [unwired: 1 out]
        n68 = call "Drive_Vi.vi"("Middle Thumb"=FALSE, "Z"=0.0, "Y"=0.15, "X"=0.0) -> ()  [unwired: 8 in]
        n69 = call <vilib>:"CTRE_Phoenix_MotorControl_Set.vi"("error in (no error)"=w135, "Output"=0.35, "Control Mode"=w132, "PhoenixMotorControlDevRef"=w134) -> ("error out"=w121:errorcluster, "PhoenixMotorControlDevRef"=w120:T9)  [unwired: 6 in]
        n70 = call <vilib>:"CTRE_Phoenix_MotorControl_Set.vi"("error in (no error)"=w137, "Output"=-0.35, "Control Mode"=w133, "PhoenixMotorControlDevRef"=w136) -> ("error out"=w118:errorcluster, "PhoenixMotorControlDevRef"=w119:T9)  [unwired: 6 in]
      }
      n71 = while {
        tunnel: w52 -> [w113]
        tunnel: w51 -> [w112]
        tunnel: w50 -> [w111]
        tunnel: w49 -> [w110]
        i -> [w108]
        stop <- w107 stop-if-true
        w116 = T13 0 items=["PercentOutput"=0, "Position"=1, "Velocity"=2, "Current"=3, "Follower"=5, "MotionProfile"=6, "MotionMagic"=7, "MotionProfileArc"=10, "Disabled"=15] ("Control Mode")
        w117 = T13 0 items=["PercentOutput"=0, "Position"=1, "Velocity"=2, "Current"=3, "Follower"=5, "MotionProfile"=6, "MotionMagic"=7, "MotionProfileArc"=10, "Disabled"=15] ("Control Mode")
        n72 = call <vilib>:"CTRE_Phoenix_MotorControl_Set.vi"("error in (no error)"=w113, "Output"=0.0, "Control Mode"=w116, "PhoenixMotorControlDevRef"=w112) -> ()  [unwired: 6 in, 2 out]
        n73 = call <vilib>:"CTRE_Phoenix_MotorControl_Set.vi"("error in (no error)"=w110, "Output"=0.0, "Control Mode"=w117, "PhoenixMotorControlDevRef"=w111) -> ()  [unwired: 6 in, 2 out]
        n74 = Greater?(x=w108, y=50) -> (0:w107:bool)
        n75 = Wait (ms)(milliseconds to wait=u32 100) -> ()  [unwired: 1 out]
      }
    }
    frame "1 Ball + Reject" {
      # "Pigeon Set"
      n76 = while {
        i -> [w496]
        stop <- w497 stop-if-true
        n77 = Wait (ms)(milliseconds to wait=u32 20) -> ()  [unwired: 1 out]
        n78 = Greater?(x=w496, y=2) -> (0:w497:bool)
        n79 = call "Drive_Vi.vi"("Middle Thumb"=TRUE, "Z"=0.0, "Y"=0.0, "X"=0.0) -> ()  [unwired: 8 in]
      }
      n80 = call <vilib>:"WPI_SwitchRefNum Registry Get.vi"("refnum name"="Intake Sensor") -> ("error out"=w317:errorcluster, "SwitchDevRef"=w316:T4)  [unwired: 9 in]
      n81 = call <vilib>:"WPI_SolenoidRefNum Registry Get.vi"("refnum name"="Intake Solenoid") -> ("error out"=w315:errorcluster, "SolenoidDevRef"=w314:T7)  [unwired: 9 in]
      n82 = call <vilib>:"CTRE_Phoenix_MotorControl_RefNumRegistryGet.vi"("refnum name"="Intake") -> ("error out"=w309:errorcluster, "PhoenixMotorControlDevRef"=w308:T9)  [unwired: 9 in]
      n83 = call <vilib>:"CTRE_Phoenix_MotorControl_RefNumRegistryGet.vi"("refnum name"="Reject") -> ("error out"=w311:errorcluster, "PhoenixMotorControlDevRef"=w310:T9)  [unwired: 9 in]
      n84 = call "Limit_Switches.vi"() -> ()  [unwired: 10 in, 2 out]
      n85 = call <vilib>:"CTRE_Phoenix_MotorControl_RefNumRegistryGet.vi"("refnum name"="Elevate") -> ("error out"=w313:errorcluster, "PhoenixMotorControlDevRef"=w312:T9)  [unwired: 9 in]
      n86 = call <vilib>:"WPI_SwitchRefNum Registry Get.vi"("refnum name"="Elevate Sensor") -> ("error out"=w319:errorcluster, "SwitchDevRef"=w318:T4)  [unwired: 9 in]
      n87 = call <vilib>:"CTRE_Phoenix_MotorControl_RefNumRegistryGet.vi"("refnum name"="Shoot") -> ("error out"=w297:errorcluster, "PhoenixMotorControlDevRef"=w296:T9)  [unwired: 9 in]
      n88 = while {
        tunnel: w319 -> [w451]
        tunnel: w318 -> [w450]
        tunnel: w317 -> [w449]
        tunnel: w316 -> [w448]
        tunnel: w315 -> [w447]
        tunnel: w314 -> [w446]
        tunnel: w313 -> [w443]
        tunnel: w312 -> [w442]
        tunnel: w311 -> [w441]
        tunnel: w310 -> [w440]
        tunnel: w309 -> [w439]
        tunnel: w308 -> [w438]
        tunnel: [w426] -> w301
        tunnel: [w425] -> w300
        tunnel: [w424] -> w299
        tunnel: [w423] -> w298
        tunnel: w297 -> [w422]
        tunnel: w296 -> [w421]
        tunnel: [w418] -> w295
        tunnel: [w417] -> w294
        tunnel: [w416] -> w287
        tunnel: [w415] -> w286
        i -> [w454]
        stop <- w455 stop-if-true
        w420 = T13 0 items=["PercentOutput"=0, "Position"=1, "Velocity"=2, "Current"=3, "Follower"=5, "MotionProfile"=6, "MotionMagic"=7, "MotionProfileArc"=10, "Disabled"=15] ("Control Mode")
        w432 = T13 0 items=["PercentOutput"=0, "Position"=1, "Velocity"=2, "Current"=3, "Follower"=5, "MotionProfile"=6, "MotionMagic"=7, "MotionProfileArc"=10, "Disabled"=15] ("Control Mode")
        w433 = T13 0 items=["PercentOutput"=0, "Position"=1, "Velocity"=2, "Current"=3, "Follower"=5, "MotionProfile"=6, "MotionMagic"=7, "MotionProfileArc"=10, "Disabled"=15] ("Control Mode")
        w434 = T13 0 items=["PercentOutput"=0, "Position"=1, "Velocity"=2, "Current"=3, "Follower"=5, "MotionProfile"=6, "MotionMagic"=7, "MotionProfileArc"=10, "Disabled"=15] ("Control Mode")
        n89 = call <vilib>:"WPI_SwitchGetLimitValue.vi"("error in (no error)"=w449, "SwitchDevRef"=w448) -> ("Switch Pressed"=w452:bool)  [unwired: 7 in, 2 out]
        n90 = call <vilib>:"WPI_SwitchGetLimitValue.vi"("error in (no error)"=w451, "SwitchDevRef"=w450) -> ("Switch Pressed"=w453:bool)  [unwired: 7 in, 2 out]
        n91 = Greater?(x=w454, y=20) -> (0:w455:bool)
        n92 = Not(x=w452) -> (.not. x?=w437:bool)
        "Intake 3" <- w437
        n93 = Not(x=w453) -> (.not. x?=w445:bool)
        "Elevate 3" <- w445
        n94 = Wait (ms)(milliseconds to wait=u32 100) -> ()  [unwired: 1 out]
        n95 = case shown="True" w445 {
          tunnel: [0.75 ("Output") w474] -> w444
          tunnel: w437 -> [_ w471]
          tunnel: [0.75 ("Output") w473] -> w436
          tunnel: [-0.1 ("Output") w472] -> w435
          tunnel: [FALSE ("Middle Thumb") w470] -> w431
          tunnel: [0.0 ("Z") w469] -> w430
          tunnel: [0.0 ("Y") w468] -> w429
          tunnel: [0.0 ("X") w467] -> w428
          tunnel: [WPI_SolenoidValue."Reverse" ("Value") w466] -> w427
          frame False {
          }
          frame True {
            n96 = case shown="False" w471 {
              tunnel: [0.75 ("Output") 0.0 ("Output")] -> w474
              tunnel: [0.75 ("Output") -0.75 ("Output")] -> w473
              tunnel: [0.0 ("Output") 0.0 ("Output")] -> w472
              tunnel: [FALSE ("Middle Thumb") FALSE ("Middle Thumb")] -> w470
              tunnel: [0.0 ("Z") 0.0 ("Z")] -> w469
              tunnel: [-0.3 ("Y") 0.0 ("Y")] -> w468
              tunnel: [0.0 ("X") 0.0 ("X")] -> w467
              tunnel: [WPI_SolenoidValue."Reverse" ("Value") WPI_SolenoidValue."Forward" ("Value")] -> w466
              frame False {
              }
              frame True {
              }
            }
          }
        }
        n97 = call-poly <vilib>:"WPI_SolenoidSet.vi"("error in (no error)"=w447, "Value"=w427, "SolenoidDevRef"=w446) -> ("error out"=w415:errorcluster, "SolenoidDevRef"=w416:T7)  [unwired: 7 in]
        n98 = call <vilib>:"CTRE_Phoenix_MotorControl_Set.vi"("error in (no error)"=w439, "Output"=w444, "Control Mode"=w432, "PhoenixMotorControlDevRef"=w438) -> ("error out"=w424:errorcluster, "PhoenixMotorControlDevRef"=w423:T9)  [unwired: 6 in]
        n99 = call <vilib>:"CTRE_Phoenix_MotorControl_Set.vi"("error in (no error)"=w441, "Output"=w436, "Control Mode"=w433, "PhoenixMotorControlDevRef"=w440) -> ()  [unwired: 6 in, 2 out]
        n100 = call <vilib>:"CTRE_Phoenix_MotorControl_Set.vi"("error in (no error)"=w443, "Output"=w435, "Control Mode"=w434, "PhoenixMotorControlDevRef"=w442) -> ("error out"=w426:errorcluster, "PhoenixMotorControlDevRef"=w425:T9)  [unwired: 6 in]
        n101 = call <vilib>:"CTRE_Phoenix_MotorControl_Set.vi"("error in (no error)"=w422, "Output"=-0.55, "Control Mode"=w420, "PhoenixMotorControlDevRef"=w421) -> ("error out"=w418:errorcluster, "PhoenixMotorControlDevRef"=w417:T9)  [unwired: 6 in]
        n102 = call "Drive_Vi.vi"("Middle Thumb"=w431, "Z"=w430, "Y"=w429, "X"=w428) -> ()  [unwired: 8 in]
      }
      n103 = call <vilib>:"WPI_SwitchRefNum Registry Get.vi"("refnum name"="Orange Limit Switch") -> ("error out"=w303:errorcluster, "SwitchDevRef"=w302:T4)  [unwired: 9 in]
      n104 = call <vilib>:"WPI_SwitchRefNum Registry Get.vi"("refnum name"="Blue Limit Switch") -> ("error out"=w305:errorcluster, "SwitchDevRef"=w304:T4)  [unwired: 9 in]
      n105 = while {
        tunnel: w295 -> [_]
        tunnel: w294 -> [_]
        tunnel: w305 -> [w412]
        tunnel: w304 -> [w411]
        tunnel: w303 -> [w410]
        tunnel: w302 -> [w409]
        tunnel: w301 -> [w388]
        tunnel: w300 -> [w387]
        tunnel: w299 -> [w378]
        tunnel: w298 -> [w379]
        tunnel: [w392] -> w293
        tunnel: [w391] -> w292
        tunnel: [w390] -> w291
        tunnel: [w389] -> w290
        tunnel: [w388] -> w289
        tunnel: [w387] -> w288
        tunnel: w287 -> [w386]
        tunnel: w286 -> [w385]
        tunnel: [w383] -> w285
        tunnel: [w382] -> w284
        tunnel: [w381] -> w283
        tunnel: [w380] -> w282
        i -> [w398]
        stop <- w397 stop-if-true
        w377 = T13 0 items=["PercentOutput"=0, "Position"=1, "Velocity"=2, "Current"=3, "Follower"=5, "MotionProfile"=6, "MotionMagic"=7, "MotionProfileArc"=10, "Disabled"=15] ("Control Mode")
        n106 = call-poly <vilib>:"WPI_SolenoidSet.vi"("error in (no error)"=w385, "Value"=WPI_SolenoidValue."Forward", "SolenoidDevRef"=w386) -> ("error out"=w382:errorcluster, "SolenoidDevRef"=w383:T7)  [unwired: 7 in]
        n107 = call <vilib>:"WPI_SwitchGetLimitValue.vi"("error in (no error)"=w410, "SwitchDevRef"=w409) -> ("error out"=w389:errorcluster, "Switch Pressed"=w408:bool, "SwitchDevRef"=w390:T4)  [unwired: 7 in]
        "Orange Limit Pressed 5" <- w408
        n108 = call <vilib>:"WPI_SwitchGetLimitValue.vi"("error in (no error)"=w412, "SwitchDevRef"=w411) -> ("error out"=w391:errorcluster, "Switch Pressed"=w407:bool, "SwitchDevRef"=w392:T4)  [unwired: 7 in]
        "Blue Limit Pressed 5" <- w407
        n109 = call-poly <vilib>:"NT Read Value.vi"("Default Value"=0.0, "Name"="/limelight-drtrain/ty") -> ("Numeric"=w402:dbl)  [unwired: 8 in, 1 out]
        "Ty 5" <- w402
        n110 = Greater?(x=w398, y=5) -> (0:w397:bool)
        n111 = call "Turret_Aim.vi"("View Button"=FALSE ("Driver Right Thumb"), "Left Trigger"=2.0, "Orange Limit Pressed"=w407, "Blue Limit Pressed"=w408, "Right Bumper"=FALSE, "Left Bumper"=FALSE) -> ()  [unwired: 6 in]
        n112 = call "Shooter_Equation.vi"("Right Trigger"=2.0, "Ty"=w402) -> ()  [unwired: 10 in]
        n113 = Wait (ms)(milliseconds to wait=u32 100) -> ()  [unwired: 1 out]
        n114 = call "Drive_Vi.vi"("Middle Thumb"=FALSE, "Z"=0.0, "Y"=0.15, "X"=0.0) -> ()  [unwired: 8 in]
        n115 = call <vilib>:"CTRE_Phoenix_MotorControl_Set.vi"("error in (no error)"=w378, "Output"=0.0, "Control Mode"=w377, "PhoenixMotorControlDevRef"=w379) -> ("error out"=w380:errorcluster, "PhoenixMotorControlDevRef"=w381:T9)  [unwired: 6 in]
      }
      n116 = while {
        tunnel: w292 -> [w373]
        tunnel: w293 -> [w372]
        tunnel: w290 -> [w371]
        tunnel: w289 -> [w358]
        tunnel: w288 -> [w357]
        tunnel: w282 -> [w356]
        tunnel: w283 -> [w355]
        tunnel: w291 -> [w346]
        tunnel: w285 -> [w345]
        tunnel: w284 -> [w344]
        tunnel: [w342] -> w281
        tunnel: [w341] -> w280
        tunnel: [w340] -> w279
        tunnel: [w339] -> w278
        i -> [w360]
        stop <- w359 stop-if-true
        w353 = T13 0 items=["PercentOutput"=0, "Position"=1, "Velocity"=2, "Current"=3, "Follower"=5, "MotionProfile"=6, "MotionMagic"=7, "MotionProfileArc"=10, "Disabled"=15] ("Control Mode")
        w354 = T13 0 items=["PercentOutput"=0, "Position"=1, "Velocity"=2, "Current"=3, "Follower"=5, "MotionProfile"=6, "MotionMagic"=7, "MotionProfileArc"=10, "Disabled"=15] ("Control Mode")
        n117 = call-poly <vilib>:"WPI_SolenoidSet.vi"("error in (no error)"=w344, "Value"=WPI_SolenoidValue."Off", "SolenoidDevRef"=w345) -> ()  [unwired: 7 in, 2 out]
        n118 = call <vilib>:"WPI_SwitchGetLimitValue.vi"("error in (no error)"=w371, "SwitchDevRef"=w346) -> ("Switch Pressed"=w370:bool)  [unwired: 7 in, 2 out]
        "Orange Limit Pressed 6" <- w370
        n119 = call <vilib>:"WPI_SwitchGetLimitValue.vi"("error in (no error)"=w373, "SwitchDevRef"=w372) -> ("Switch Pressed"=w369:bool)  [unwired: 7 in, 2 out]
        "Blue Limit Pressed 6" <- w369
        n120 = call-poly <vilib>:"NT Read Value.vi"("Default Value"=0.0, "Name"="/limelight-drtrain/ty") -> ("Numeric"=w364:dbl)  [unwired: 8 in, 1 out]
        "Ty 6" <- w364
        n121 = Greater?(x=w360, y=50) -> (0:w359:bool)
        n122 = call "Turret_Aim.vi"("View Button"=FALSE ("Driver Right Thumb"), "Left Trigger"=2.0, "Orange Limit Pressed"=w369, "Blue Limit Pressed"=w370, "Right Bumper"=FALSE, "Left Bumper"=FALSE) -> ()  [unwired: 6 in]
        n123 = call "Shooter_Equation.vi"("Right Trigger"=2.0, "Ty"=w364) -> ()  [unwired: 10 in]
        n124 = Wait (ms)(milliseconds to wait=u32 100) -> ()  [unwired: 1 out]
        n125 = call "Drive_Vi.vi"("Middle Thumb"=FALSE, "Z"=0.0, "Y"=0.15, "X"=0.0) -> ()  [unwired: 8 in]
        n126 = call <vilib>:"CTRE_Phoenix_MotorControl_Set.vi"("error in (no error)"=w356, "Output"=0.35, "Control Mode"=w353, "PhoenixMotorControlDevRef"=w355) -> ("error out"=w342:errorcluster, "PhoenixMotorControlDevRef"=w341:T9)  [unwired: 6 in]
        n127 = call <vilib>:"CTRE_Phoenix_MotorControl_Set.vi"("error in (no error)"=w358, "Output"=-0.35, "Control Mode"=w354, "PhoenixMotorControlDevRef"=w357) -> ("error out"=w339:errorcluster, "PhoenixMotorControlDevRef"=w340:T9)  [unwired: 6 in]
      }
      n128 = while {
        tunnel: w281 -> [w334]
        tunnel: w280 -> [w333]
        tunnel: w279 -> [w332]
        tunnel: w278 -> [w331]
        i -> [w329]
        stop <- w328 stop-if-true
        w337 = T13 0 items=["PercentOutput"=0, "Position"=1, "Velocity"=2, "Current"=3, "Follower"=5, "MotionProfile"=6, "MotionMagic"=7, "MotionProfileArc"=10, "Disabled"=15] ("Control Mode")
        w338 = T13 0 items=["PercentOutput"=0, "Position"=1, "Velocity"=2, "Current"=3, "Follower"=5, "MotionProfile"=6, "MotionMagic"=7, "MotionProfileArc"=10, "Disabled"=15] ("Control Mode")
        n129 = call <vilib>:"CTRE_Phoenix_MotorControl_Set.vi"("error in (no error)"=w334, "Output"=0.0, "Control Mode"=w337, "PhoenixMotorControlDevRef"=w333) -> ()  [unwired: 6 in, 2 out]
        n130 = call <vilib>:"CTRE_Phoenix_MotorControl_Set.vi"("error in (no error)"=w331, "Output"=0.0, "Control Mode"=w338, "PhoenixMotorControlDevRef"=w332) -> ()  [unwired: 6 in, 2 out]
        n131 = Greater?(x=w329, y=50) -> (0:w328:bool)
        n132 = Wait (ms)(milliseconds to wait=u32 100) -> ()  [unwired: 1 out]
      }
    }
    frame "2 Ball" {
      # "Pigeon Set"
      n133 = while {
        i -> [w770]
        stop <- w771 stop-if-true
        n134 = Wait (ms)(milliseconds to wait=u32 20) -> ()  [unwired: 1 out]
        n135 = Greater?(x=w770, y=2) -> (0:w771:bool)
        n136 = call "Drive_Vi.vi"("Middle Thumb"=TRUE, "Z"=0.0, "Y"=0.0, "X"=0.0) -> ()  [unwired: 8 in]
      }
      n137 = call <vilib>:"WPI_SwitchRefNum Registry Get.vi"("refnum name"="Intake Sensor") -> ("error out"=w545:errorcluster, "SwitchDevRef"=w544:T4)  [unwired: 9 in]
      n138 = call <vilib>:"CTRE_Phoenix_MotorControl_RefNumRegistryGet.vi"("refnum name"="Intake") -> ("error out"=w539:errorcluster, "PhoenixMotorControlDevRef"=w538:T9)  [unwired: 9 in]
      n139 = call <vilib>:"CTRE_Phoenix_MotorControl_RefNumRegistryGet.vi"("refnum name"="Intake Actuate") -> ("error out"=w514:errorcluster, "PhoenixMotorControlDevRef"=w513:T9)  [unwired: 9 in]
      n140 = call <vilib>:"CTRE_Phoenix_MotorControl_RefNumRegistryGet.vi"("refnum name"="Reject") -> ("error out"=w541:errorcluster, "PhoenixMotorControlDevRef"=w540:T9)  [unwired: 9 in]
      n141 = call "Limit_Switches.vi"() -> ()  [unwired: 10 in, 2 out]
      n142 = call <vilib>:"CTRE_Phoenix_MotorControl_RefNumRegistryGet.vi"("refnum name"="Elevate") -> ("error out"=w543:errorcluster, "PhoenixMotorControlDevRef"=w542:T9)  [unwired: 9 in]
      n143 = call <vilib>:"WPI_SwitchRefNum Registry Get.vi"("refnum name"="Elevate Sensor") -> ("error out"=w547:errorcluster, "SwitchDevRef"=w546:T4)  [unwired: 9 in]
      n144 = call <vilib>:"CTRE_Phoenix_MotorControl_RefNumRegistryGet.vi"("refnum name"="Shoot") -> ("error out"=w527:errorcluster, "PhoenixMotorControlDevRef"=w526:T9)  [unwired: 9 in]
      n145 = while {
        tunnel: w547 -> [w729]
        tunnel: w546 -> [w728]
        tunnel: w545 -> [w727]
        tunnel: w544 -> [w726]
        tunnel: w543 -> [w723]
        tunnel: w542 -> [w722]
        tunnel: w541 -> [w721]
        tunnel: w540 -> [w720]
        tunnel: w539 -> [w719]
        tunnel: w538 -> [w718]
        tunnel: [w707] -> w531
        tunnel: [w706] -> w530
        tunnel: [w705] -> w529
        tunnel: [w704] -> w528
        tunnel: w527 -> [w703]
        tunnel: w526 -> [w702]
        tunnel: [w699] -> w525
        tunnel: [w698] -> w524
        tunnel: w514 -> [w697]
        tunnel: w513 -> [w696]
        tunnel: [w693] -> w512
        tunnel: [w692] -> w511
        i -> [w732]
        stop <- w733 stop-if-true
        w695 = T13 0 items=["PercentOutput"=0, "Position"=1, "Velocity"=2, "Current"=3, "Follower"=5, "MotionProfile"=6, "MotionMagic"=7, "MotionProfileArc"=10, "Disabled"=15] ("Control Mode")
        w701 = T13 0 items=["PercentOutput"=0, "Position"=1, "Velocity"=2, "Current"=3, "Follower"=5, "MotionProfile"=6, "MotionMagic"=7, "MotionProfileArc"=10, "Disabled"=15] ("Control Mode")
        w712 = T13 0 items=["PercentOutput"=0, "Position"=1, "Velocity"=2, "Current"=3, "Follower"=5, "MotionProfile"=6, "MotionMagic"=7, "MotionProfileArc"=10, "Disabled"=15] ("Control Mode")
        w713 = T13 0 items=["PercentOutput"=0, "Position"=1, "Velocity"=2, "Current"=3, "Follower"=5, "MotionProfile"=6, "MotionMagic"=7, "MotionProfileArc"=10, "Disabled"=15] ("Control Mode")
        w714 = T13 0 items=["PercentOutput"=0, "Position"=1, "Velocity"=2, "Current"=3, "Follower"=5, "MotionProfile"=6, "MotionMagic"=7, "MotionProfileArc"=10, "Disabled"=15] ("Control Mode")
        n146 = call <vilib>:"CTRE_Phoenix_MotorControl_Set.vi"("error in (no error)"=w697, "Output"=-0.2, "Control Mode"=w695, "PhoenixMotorControlDevRef"=w696) -> ("error out"=w692:errorcluster, "PhoenixMotorControlDevRef"=w693:T9)  [unwired: 6 in]
        n147 = global write "AutonBoolean.vi" "Boolean"(TRUE ("Boolean")) -> ()
        n148 = call <vilib>:"WPI_SwitchGetLimitValue.vi"("error in (no error)"=w727, "SwitchDevRef"=w726) -> ("Switch Pressed"=w730:bool)  [unwired: 7 in, 2 out]
        n149 = call <vilib>:"WPI_SwitchGetLimitValue.vi"("error in (no error)"=w729, "SwitchDevRef"=w728) -> ("Switch Pressed"=w731:bool)  [unwired: 7 in, 2 out]
        n150 = Greater?(x=w732, y=20) -> (0:w733:bool)
        n151 = Not(x=w730) -> (.not. x?=w717:bool)
        "Intake" <- w717
        n152 = Not(x=w731) -> (.not. x?=w725:bool)
        "Elevate" <- w725
        n153 = Wait (ms)(milliseconds to wait=u32 100) -> ()  [unwired: 1 out]
        n154 = case shown="True" w725 {
          tunnel: [0.8 ("Output") w750] -> w724
          tunnel: w717 -> [_ w747]
          tunnel: [0.75 ("Output") w749] -> w716
          tunnel: [-0.1 ("Output") w748] -> w715
          tunnel: [FALSE ("Middle Thumb") w746] -> w711
          tunnel: [0.0 ("Z") w745] -> w710
          tunnel: [0.0 ("Y") w744] -> w709
          tunnel: [0.0 ("X") w743] -> w708
          frame False {
          }
          frame True {
            n155 = case shown="False" w747 {
              tunnel: [1.0 ("Output") 0.0 ("Output")] -> w750
              tunnel: [0.0 ("Output") 0.0 ("Output")] -> w749
              tunnel: [0.0 ("Output") 0.0 ("Output")] -> w748
              tunnel: [FALSE ("Middle Thumb") FALSE ("Middle Thumb")] -> w746
              tunnel: [0.0 ("Z") 0.0 ("Z")] -> w745
              tunnel: [-0.3 ("Y") 0.0 ("Y")] -> w744
              tunnel: [0.0 ("X") 0.0 ("X")] -> w743
              frame False {
              }
              frame True {
              }
            }
          }
        }
        n156 = call <vilib>:"CTRE_Phoenix_MotorControl_Set.vi"("error in (no error)"=w719, "Output"=w724, "Control Mode"=w712, "PhoenixMotorControlDevRef"=w718) -> ("error out"=w705:errorcluster, "PhoenixMotorControlDevRef"=w704:T9)  [unwired: 6 in]
        n157 = call <vilib>:"CTRE_Phoenix_MotorControl_Set.vi"("error in (no error)"=w721, "Output"=w716, "Control Mode"=w713, "PhoenixMotorControlDevRef"=w720) -> ()  [unwired: 6 in, 2 out]
        n158 = call <vilib>:"CTRE_Phoenix_MotorControl_Set.vi"("error in (no error)"=w723, "Output"=w715, "Control Mode"=w714, "PhoenixMotorControlDevRef"=w722) -> ("error out"=w707:errorcluster, "PhoenixMotorControlDevRef"=w706:T9)  [unwired: 6 in]
        n159 = call <vilib>:"CTRE_Phoenix_MotorControl_Set.vi"("error in (no error)"=w703, "Output"=-0.55, "Control Mode"=w701, "PhoenixMotorControlDevRef"=w702) -> ("error out"=w699:errorcluster, "PhoenixMotorControlDevRef"=w698:T9)  [unwired: 6 in]
        n160 = call "Drive_Vi.vi"("Middle Thumb"=w711, "Z"=w710, "Y"=w709, "X"=w708) -> ()  [unwired: 8 in]
      }
      n161 = call <vilib>:"WPI_SwitchRefNum Registry Get.vi"("refnum name"="Orange Limit Switch") -> ("error out"=w533:errorcluster, "SwitchDevRef"=w532:T4)  [unwired: 9 in]
      n162 = call <vilib>:"WPI_SwitchRefNum Registry Get.vi"("refnum name"="Blue Limit Switch") -> ("error out"=w535:errorcluster, "SwitchDevRef"=w534:T4)  [unwired: 9 in]
      n163 = while {
        tunnel: w525 -> [_]
        tunnel: w524 -> [_]
        tunnel: w535 -> [w688]
        tunnel: w534 -> [w687]
        tunnel: w533 -> [w686]
        tunnel: w532 -> [w685]
        tunnel: w531 -> [w664]
        tunnel: w530 -> [w663]
        tunnel: w529 -> [w659]
        tunnel: w528 -> [w660]
        tunnel: [w668] -> w523
        tunnel: [w667] -> w522
        tunnel: [w666] -> w521
        tunnel: [w665] -> w520
        tunnel: [w664] -> w519
        tunnel: [w663] -> w518
        tunnel: [w662] -> w517
        tunnel: [w661] -> w516
        tunnel: w512 -> [w654]
        tunnel: w511 -> [w653]
        i -> [w674]
        stop <- w673 stop-if-true
        w656 = T13 0 items=["PercentOutput"=0, "Position"=1, "Velocity"=2, "Current"=3, "Follower"=5, "MotionProfile"=6, "MotionMagic"=7, "MotionProfileArc"=10, "Disabled"=15] ("Control Mode")
        w658 = T13 0 items=["PercentOutput"=0, "Position"=1, "Velocity"=2, "Current"=3, "Follower"=5, "MotionProfile"=6, "MotionMagic"=7, "MotionProfileArc"=10, "Disabled"=15] ("Control Mode")
        n164 = call <vilib>:"CTRE_Phoenix_MotorControl_Set.vi"("error in (no error)"=w653, "Output"=0.0, "Control Mode"=w656, "PhoenixMotorControlDevRef"=w654) -> ()  [unwired: 6 in, 2 out]
        n165 = call <vilib>:"WPI_SwitchGetLimitValue.vi"("error in (no error)"=w686, "SwitchDevRef"=w685) -> ("error out"=w665:errorcluster, "Switch Pressed"=w684:bool, "SwitchDevRef"=w666:T4)  [unwired: 7 in]
        "Orange Limit Pressed" <- w684
        n166 = call <vilib>:"WPI_SwitchGetLimitValue.vi"("error in (no error)"=w688, "SwitchDevRef"=w687) -> ("error out"=w667:errorcluster, "Switch Pressed"=w683:bool, "SwitchDevRef"=w668:T4)  [unwired: 7 in]
        "Blue Limit Pressed" <- w683
        n167 = call-poly <vilib>:"NT Read Value.vi"("Default Value"=0.0, "Name"="/limelight-drtrain/ty") -> ("Numeric"=w678:dbl)  [unwired: 8 in, 1 out]
        "Ty" <- w678
        n168 = global write "AutonBoolean.vi" "Boolean"(FALSE ("Boolean")) -> ()
        n169 = Greater?(x=w674, y=5) -> (0:w673:bool)
        n170 = call "Turret_Aim.vi"("View Button"=FALSE ("Driver Right Thumb"), "Left Trigger"=2.0, "Orange Limit Pressed"=w683, "Blue Limit Pressed"=w684, "Right Bumper"=FALSE, "Left Bumper"=FALSE) -> ()  [unwired: 6 in]
        n171 = call "Shooter_Equation.vi"("Right Trigger"=2.0, "Ty"=w678) -> ()  [unwired: 10 in]
        n172 = Wait (ms)(milliseconds to wait=u32 100) -> ()  [unwired: 1 out]
        n173 = call "Drive_Vi.vi"("Middle Thumb"=FALSE, "Z"=0.0, "Y"=0.15, "X"=0.0) -> ()  [unwired: 8 in]
        n174 = call <vilib>:"CTRE_Phoenix_MotorControl_Set.vi"("error in (no error)"=w659, "Output"=0.0, "Control Mode"=w658, "PhoenixMotorControlDevRef"=w660) -> ("error out"=w661:errorcluster, "PhoenixMotorControlDevRef"=w662:T9)  [unwired: 6 in]
      }
      n175 = while {
        tunnel: w522 -> [w649]
        tunnel: w523 -> [w648]
        tunnel: w520 -> [w647]
        tunnel: w519 -> [w634]
        tunnel: w518 -> [w633]
        tunnel: w516 -> [w632]
        tunnel: w517 -> [w631]
        tunnel: w521 -> [w622]
        tunnel: [w621] -> w509
        tunnel: [w620] -> w510
        tunnel: [w619] -> w508
        tunnel: [w618] -> w507
        i -> [w636]
        stop <- w635 stop-if-true
        w629 = T13 0 items=["PercentOutput"=0, "Position"=1, "Velocity"=2, "Current"=3, "Follower"=5, "MotionProfile"=6, "MotionMagic"=7, "MotionProfileArc"=10, "Disabled"=15] ("Control Mode")
        w630 = T13 0 items=["PercentOutput"=0, "Position"=1, "Velocity"=2, "Current"=3, "Follower"=5, "MotionProfile"=6, "MotionMagic"=7, "MotionProfileArc"=10, "Disabled"=15] ("Control Mode")
        n176 = call <vilib>:"WPI_SwitchGetLimitValue.vi"("error in (no error)"=w647, "SwitchDevRef"=w622) -> ("Switch Pressed"=w646:bool)  [unwired: 7 in, 2 out]
        "Orange Limit Pressed 2" <- w646
        n177 = call <vilib>:"WPI_SwitchGetLimitValue.vi"("error in (no error)"=w649, "SwitchDevRef"=w648) -> ("Switch Pressed"=w645:bool)  [unwired: 7 in, 2 out]
        "Blue Limit Pressed 2" <- w645
        n178 = call-poly <vilib>:"NT Read Value.vi"("Default Value"=0.0, "Name"="/limelight-drtrain/ty") -> ("Numeric"=w640:dbl)  [unwired: 8 in, 1 out]
        "Ty 2" <- w640
        n179 = Greater?(x=w636, y=50) -> (0:w635:bool)
        n180 = call "Turret_Aim.vi"("View Button"=FALSE ("Driver Right Thumb"), "Left Trigger"=2.0, "Orange Limit Pressed"=w645, "Blue Limit Pressed"=w646, "Right Bumper"=FALSE, "Left Bumper"=FALSE) -> ()  [unwired: 6 in]
        n181 = call "Shooter_Equation.vi"("Right Trigger"=2.0, "Ty"=w640) -> ()  [unwired: 10 in]
        n182 = Wait (ms)(milliseconds to wait=u32 100) -> ()  [unwired: 1 out]
        n183 = call "Drive_Vi.vi"("Middle Thumb"=FALSE, "Z"=0.0, "Y"=0.15, "X"=0.0) -> ()  [unwired: 8 in]
        n184 = call <vilib>:"CTRE_Phoenix_MotorControl_Set.vi"("error in (no error)"=w632, "Output"=0.35, "Control Mode"=w629, "PhoenixMotorControlDevRef"=w631) -> ("error out"=w621:errorcluster, "PhoenixMotorControlDevRef"=w620:T9)  [unwired: 6 in]
        n185 = call <vilib>:"CTRE_Phoenix_MotorControl_Set.vi"("error in (no error)"=w634, "Output"=-0.35, "Control Mode"=w630, "PhoenixMotorControlDevRef"=w633) -> ("error out"=w618:errorcluster, "PhoenixMotorControlDevRef"=w619:T9)  [unwired: 6 in]
      }
      n186 = while {
        tunnel: w507 -> [w593]
        tunnel: w508 -> [w592]
        tunnel: w509 -> [w591]
        tunnel: w510 -> [w590]
        tunnel: [w581] -> w505
        tunnel: [w580] -> w506
        tunnel: [w579] -> w504
        tunnel: [w578] -> w503
        i -> [w595]
        stop <- w594 stop-if-true
        w588 = T13 0 items=["PercentOutput"=0, "Position"=1, "Velocity"=2, "Current"=3, "Follower"=5, "MotionProfile"=6, "MotionMagic"=7, "MotionProfileArc"=10, "Disabled"=15] ("Control Mode")
        w589 = T13 0 items=["PercentOutput"=0, "Position"=1, "Velocity"=2, "Current"=3, "Follower"=5, "MotionProfile"=6, "MotionMagic"=7, "MotionProfileArc"=10, "Disabled"=15] ("Control Mode")
        n187 = call-poly <vilib>:"NT Read Value.vi"("Default Value"=0.0, "Name"="/limelight-drtrain/ty") -> ("Numeric"=w599:dbl)  [unwired: 8 in, 1 out]
        "Ty 23" <- w599
        n188 = Greater?(x=w595, y=10) -> (0:w594:bool)
        n189 = call "Shooter_Equation.vi"("Right Trigger"=0.0, "Ty"=w599) -> ()  [unwired: 10 in]
        n190 = Wait (ms)(milliseconds to wait=u32 112) -> ()  [unwired: 1 out]
        n191 = call "Drive_Vi.vi"("Middle Thumb"=FALSE, "Z"=0.35, "Y"=0.0, "X"=0.0) -> ()  [unwired: 8 in]
        n192 = call <vilib>:"CTRE_Phoenix_MotorControl_Set.vi"("error in (no error)"=w591, "Output"=0.35, "Control Mode"=w588, "PhoenixMotorControlDevRef"=w590) -> ("error out"=w581:errorcluster, "PhoenixMotorControlDevRef"=w580:T9)  [unwired: 6 in]
        n193 = call <vilib>:"CTRE_Phoenix_MotorControl_Set.vi"("error in (no error)"=w593, "Output"=-0.35, "Control Mode"=w589, "PhoenixMotorControlDevRef"=w592) -> ("error out"=w578:errorcluster, "PhoenixMotorControlDevRef"=w579:T9)  [unwired: 6 in]
      }
      n194 = while {
        tunnel: w503 -> [w569]
        tunnel: w504 -> [w568]
        tunnel: w505 -> [w567]
        tunnel: w506 -> [w566]
        tunnel: [w557] -> w500
        tunnel: [w556] -> w502
        tunnel: [w555] -> w501
        tunnel: [w554] -> w499
        i -> [w571]
        stop <- w570 stop-if-true
        w564 = T13 0 items=["PercentOutput"=0, "Position"=1, "Velocity"=2, "Current"=3, "Follower"=5, "MotionProfile"=6, "MotionMagic"=7, "MotionProfileArc"=10, "Disabled"=15] ("Control Mode")
        w565 = T13 0 items=["PercentOutput"=0, "Position"=1, "Velocity"=2, "Current"=3, "Follower"=5, "MotionProfile"=6, "MotionMagic"=7, "MotionProfileArc"=10, "Disabled"=15] ("Control Mode")
        n195 = call-poly <vilib>:"NT Read Value.vi"("Default Value"=0.0, "Name"="/limelight-drtrain/ty") -> ("Numeric"=w575:dbl)  [unwired: 8 in, 1 out]
        "Ty 24" <- w575
        n196 = Greater?(x=w571, y=2) -> (0:w570:bool)
        n197 = call "Shooter_Equation.vi"("Right Trigger"=0.0, "Ty"=w575) -> ()  [unwired: 10 in]
        n198 = Wait (ms)(milliseconds to wait=u32 20) -> ()  [unwired: 1 out]
        n199 = call "Drive_Vi.vi"("Middle Thumb"=TRUE, "Z"=0.0, "Y"=0.0, "X"=0.0) -> ()  [unwired: 8 in]
        n200 = call <vilib>:"CTRE_Phoenix_MotorControl_Set.vi"("error in (no error)"=w567, "Output"=0.35, "Control Mode"=w564, "PhoenixMotorControlDevRef"=w566) -> ("error out"=w557:errorcluster, "PhoenixMotorControlDevRef"=w556:T9)  [unwired: 6 in]
        n201 = call <vilib>:"CTRE_Phoenix_MotorControl_Set.vi"("error in (no error)"=w569, "Output"=-0.35, "Control Mode"=w565, "PhoenixMotorControlDevRef"=w568) -> ("error out"=w554:errorcluster, "PhoenixMotorControlDevRef"=w555:T9)  [unwired: 6 in]
      }
      n202 = while {
        tunnel: w500 -> [w613]
        tunnel: w502 -> [w612]
        tunnel: w501 -> [w611]
        tunnel: w499 -> [w610]
        i -> [w608]
        stop <- w607 stop-if-true
        w616 = T13 0 items=["PercentOutput"=0, "Position"=1, "Velocity"=2, "Current"=3, "Follower"=5, "MotionProfile"=6, "MotionMagic"=7, "MotionProfileArc"=10, "Disabled"=15] ("Control Mode")
        w617 = T13 0 items=["PercentOutput"=0, "Position"=1, "Velocity"=2, "Current"=3, "Follower"=5, "MotionProfile"=6, "MotionMagic"=7, "MotionProfileArc"=10, "Disabled"=15] ("Control Mode")
        n203 = call <vilib>:"CTRE_Phoenix_MotorControl_Set.vi"("error in (no error)"=w613, "Output"=0.0, "Control Mode"=w616, "PhoenixMotorControlDevRef"=w612) -> ()  [unwired: 6 in, 2 out]
        n204 = call <vilib>:"CTRE_Phoenix_MotorControl_Set.vi"("error in (no error)"=w610, "Output"=0.0, "Control Mode"=w617, "PhoenixMotorControlDevRef"=w611) -> ()  [unwired: 6 in, 2 out]
        n205 = call "Drive_Vi.vi"("Middle Thumb"=FALSE, "Z"=0.0, "Y"=0.0, "X"=0.0) -> ()  [unwired: 8 in]
        n206 = Greater?(x=w608, y=50) -> (0:w607:bool)
        n207 = Wait (ms)(milliseconds to wait=u32 100) -> ()  [unwired: 1 out]
      }
    }
    frame "Drive Test" {
      # "Get limelight position and shooter started up"
      # "Driving backwards, put arms down and running intake to get ball"
      n208 = call <vilib>:"CTRE_Phoenix_MotorControl_RefNumRegistryGet.vi"("refnum name"="Intake") -> ("error out"=w774:errorcluster, "PhoenixMotorControlDevRef"=w776:T9)  [unwired: 9 in]
      n209 = while {
        tunnel: [w783] -> w775
        tunnel: w776 -> [w783]
        tunnel: [w782] -> w773
        tunnel: w774 -> [w782]
        i -> [w789]
        stop <- w790 stop-if-true
        n210 = Wait (ms)(milliseconds to wait=u32 20) -> ()  [unwired: 1 out]
        n211 = Greater?(x=w789, y=2) -> (0:w790:bool)
        n212 = call "Drive_Vi.vi"("Middle Thumb"=TRUE, "Z"=0.0, "Y"=0.0, "X"=0.0) -> ()  [unwired: 8 in]
      }
      n213 = while {
        tunnel: w775 -> [w823]
        tunnel: w773 -> [w822]
        tunnel: [w821] -> w780
        tunnel: [w820] -> w779
        i -> [w830]
        stop <- w829 stop-if-true
        w819 = T13 0 items=["PercentOutput"=0, "Position"=1, "Velocity"=2, "Current"=3, "Follower"=5, "MotionProfile"=6, "MotionMagic"=7, "MotionProfileArc"=10, "Disabled"=15] ("Control Mode")
        # "-0.186"
        # "-0.944"
        # ".135"
        n214 = call "Drive_Vi.vi"("Middle Thumb"=FALSE, "Z"=0.0, "Y"=-0.5, "X"=0.0) -> ()  [unwired: 8 in]
        n215 = call <vilib>:"CTRE_Phoenix_MotorControl_Set.vi"("error in (no error)"=w822, "Output"=0.0, "Control Mode"=w819, "PhoenixMotorControlDevRef"=w823) -> ("error out"=w820:errorcluster, "PhoenixMotorControlDevRef"=w821:T9)  [unwired: 6 in]
        n216 = Greater?(x=w830, y=20) -> (0:w829:bool)
        n217 = Wait (ms)(milliseconds to wait=u32 100) -> ()  [unwired: 1 out]
      }
      n218 = while {
        tunnel: w780 -> [w809]
        tunnel: w779 -> [w808]
        tunnel: [w807] -> w778
        tunnel: [w806] -> w777
        i -> [w816]
        stop <- w815 stop-if-true
        w805 = T13 0 items=["PercentOutput"=0, "Position"=1, "Velocity"=2, "Current"=3, "Follower"=5, "MotionProfile"=6, "MotionMagic"=7, "MotionProfileArc"=10, "Disabled"=15] ("Control Mode")
        # "-0.186"
        # "-0.944"
        # ".135"
        n219 = call "Drive_Vi.vi"("Middle Thumb"=FALSE, "Z"=0.0, "Y"=0.15, "X"=0.0) -> ()  [unwired: 8 in]
        n220 = Greater?(x=w816, y=5) -> (0:w815:bool)
        n221 = call <vilib>:"CTRE_Phoenix_MotorControl_Set.vi"("error in (no error)"=w808, "Output"=0.0, "Control Mode"=w805, "PhoenixMotorControlDevRef"=w809) -> ("error out"=w806:errorcluster, "PhoenixMotorControlDevRef"=w807:T9)  [unwired: 6 in]
        n222 = Wait (ms)(milliseconds to wait=u32 100) -> ()  [unwired: 1 out]
      }
      n223 = while {
        tunnel: w778 -> [w795]
        tunnel: w777 -> [w794]
        i -> [w802]
        stop <- w801 stop-if-true
        w793 = T13 0 items=["PercentOutput"=0, "Position"=1, "Velocity"=2, "Current"=3, "Follower"=5, "MotionProfile"=6, "MotionMagic"=7, "MotionProfileArc"=10, "Disabled"=15] ("Control Mode")
        # "-0.186"
        # "-0.944"
        # ".135"
        n224 = call "Drive_Vi.vi"("Middle Thumb"=FALSE, "Z"=0.0, "Y"=0.0, "X"=0.0) -> ()  [unwired: 8 in]
        n225 = Greater?(x=w802, y=20) -> (0:w801:bool)
        n226 = call <vilib>:"CTRE_Phoenix_MotorControl_Set.vi"("error in (no error)"=w794, "Output"=0.0, "Control Mode"=w793, "PhoenixMotorControlDevRef"=w795) -> ()  [unwired: 6 in, 2 out]
        n227 = Wait (ms)(milliseconds to wait=u32 100) -> ()  [unwired: 1 out]
      }
    }
    frame "4 Ball" {
      # "Pigeon Set"
      n228 = while {
        i -> [w1215]
        stop <- w1216 stop-if-true
        n229 = Wait (ms)(milliseconds to wait=u32 20) -> ()  [unwired: 1 out]
        n230 = Greater?(x=w1215, y=2) -> (0:w1216:bool)
        n231 = call "Drive_Vi.vi"("Middle Thumb"=TRUE, "Z"=0.0, "Y"=0.0, "X"=0.0) -> ()  [unwired: 8 in]
      }
      n232 = call <vilib>:"WPI_SwitchRefNum Registry Get.vi"("refnum name"="Intake Sensor") -> ("error out"=w892:errorcluster, "SwitchDevRef"=w891:T4)  [unwired: 9 in]
      n233 = call <vilib>:"CTRE_Phoenix_MotorControl_RefNumRegistryGet.vi"("refnum name"="Intake") -> ("error out"=w886:errorcluster, "PhoenixMotorControlDevRef"=w885:T9)  [unwired: 9 in]
      n234 = call <vilib>:"CTRE_Phoenix_MotorControl_RefNumRegistryGet.vi"("refnum name"="Reject") -> ("error out"=w888:errorcluster, "PhoenixMotorControlDevRef"=w887:T9)  [unwired: 9 in]
      n235 = call "Limit_Switches.vi"() -> ()  [unwired: 10 in, 2 out]
      n236 = call <vilib>:"CTRE_Phoenix_MotorControl_RefNumRegistryGet.vi"("refnum name"="Elevate") -> ("error out"=w890:errorcluster, "PhoenixMotorControlDevRef"=w889:T9)  [unwired: 9 in]
      n237 = call <vilib>:"WPI_SwitchRefNum Registry Get.vi"("refnum name"="Elevate Sensor") -> ("error out"=w894:errorcluster, "SwitchDevRef"=w893:T4)  [unwired: 9 in]
      n238 = call <vilib>:"CTRE_Phoenix_MotorControl_RefNumRegistryGet.vi"("refnum name"="Shoot") -> ("error out"=w874:errorcluster, "PhoenixMotorControlDevRef"=w873:T9)  [unwired: 9 in]
      n239 = call <vilib>:"CTRE_Phoenix_MotorControl_RefNumRegistryGet.vi"("refnum name"="Intake Actuate") -> ("error out"=w840:errorcluster, "PhoenixMotorControlDevRef"=w841:T9)  [unwired: 9 in]
      n240 = while {
        tunnel: w894 -> [w1174]
        tunnel: w893 -> [w1173]
        tunnel: w892 -> [w1172]
        tunnel: w891 -> [w1171]
        tunnel: w890 -> [w1168]
        tunnel: w889 -> [w1167]
        tunnel: w888 -> [w1166]
        tunnel: w887 -> [w1165]
        tunnel: w886 -> [w1164]
        tunnel: w885 -> [w1163]
        tunnel: [w1152] -> w878
        tunnel: [w1151] -> w877
        tunnel: [w1150] -> w876
        tunnel: [w1149] -> w875
        tunnel: w874 -> [w1148]
        tunnel: w873 -> [w1147]
        tunnel: [w1144] -> w872
        tunnel: [w1143] -> w871
        i -> [w1177]
        stop <- w1178 stop-if-true
        w1146 = T13 0 items=["PercentOutput"=0, "Position"=1, "Velocity"=2, "Current"=3, "Follower"=5, "MotionProfile"=6, "MotionMagic"=7, "MotionProfileArc"=10, "Disabled"=15] ("Control Mode")
        w1157 = T13 0 items=["PercentOutput"=0, "Position"=1, "Velocity"=2, "Current"=3, "Follower"=5, "MotionProfile"=6, "MotionMagic"=7, "MotionProfileArc"=10, "Disabled"=15] ("Control Mode")
        w1158 = T13 0 items=["PercentOutput"=0, "Position"=1, "Velocity"=2, "Current"=3, "Follower"=5, "MotionProfile"=6, "MotionMagic"=7, "MotionProfileArc"=10, "Disabled"=15] ("Control Mode")
        w1159 = T13 0 items=["PercentOutput"=0, "Position"=1, "Velocity"=2, "Current"=3, "Follower"=5, "MotionProfile"=6, "MotionMagic"=7, "MotionProfileArc"=10, "Disabled"=15] ("Control Mode")
        n241 = call <vilib>:"WPI_SwitchGetLimitValue.vi"("error in (no error)"=w1172, "SwitchDevRef"=w1171) -> ("Switch Pressed"=w1175:bool)  [unwired: 7 in, 2 out]
        n242 = call <vilib>:"WPI_SwitchGetLimitValue.vi"("error in (no error)"=w1174, "SwitchDevRef"=w1173) -> ("Switch Pressed"=w1176:bool)  [unwired: 7 in, 2 out]
        n243 = Greater?(x=w1177, y=20) -> (0:w1178:bool)
        n244 = Not(x=w1175) -> (.not. x?=w1162:bool)
        "Intake 2" <- w1162
        n245 = Not(x=w1176) -> (.not. x?=w1170:bool)
        "Elevate 2" <- w1170
        n246 = Wait (ms)(milliseconds to wait=u32 100) -> ()  [unwired: 1 out]
        n247 = case shown="True" w1170 {
          tunnel: [0.75 ("Output") w1195] -> w1169
          tunnel: w1162 -> [_ w1192]
          tunnel: [0.75 ("Output") w1194] -> w1161
          tunnel: [-0.1 ("Output") w1193] -> w1160
          tunnel: [FALSE ("Middle Thumb") w1191] -> w1156
          tunnel: [0.0 ("Z") w1190] -> w1155
          tunnel: [0.0 ("Y") w1189] -> w1154
          tunnel: [0.0 ("X") w1188] -> w1153
          frame False {
            (unwired) WPI_SolenoidValue."Reverse" ("Value")
          }
          frame True {
            n248 = case shown="False" w1192 {
              tunnel: [0.75 ("Output") 0.0 ("Output")] -> w1195
              tunnel: [0.0 ("Output") 0.0 ("Output")] -> w1194
              tunnel: [0.0 ("Output") 0.0 ("Output")] -> w1193
              tunnel: [FALSE ("Middle Thumb") FALSE ("Middle Thumb")] -> w1191
              tunnel: [0.0 ("Z") 0.0 ("Z")] -> w1190
              tunnel: [-0.3 ("Y") 0.0 ("Y")] -> w1189
              tunnel: [0.0 ("X") 0.0 ("X")] -> w1188
              frame False {
              }
              frame True {
                (unwired) WPI_SolenoidValue."Forward" ("Value")
              }
            }
          }
        }
        n249 = call <vilib>:"CTRE_Phoenix_MotorControl_Set.vi"("error in (no error)"=w1164, "Output"=w1169, "Control Mode"=w1157, "PhoenixMotorControlDevRef"=w1163) -> ("error out"=w1150:errorcluster, "PhoenixMotorControlDevRef"=w1149:T9)  [unwired: 6 in]
        n250 = call <vilib>:"CTRE_Phoenix_MotorControl_Set.vi"("error in (no error)"=w1166, "Output"=w1161, "Control Mode"=w1158, "PhoenixMotorControlDevRef"=w1165) -> ()  [unwired: 6 in, 2 out]
        n251 = call <vilib>:"CTRE_Phoenix_MotorControl_Set.vi"("error in (no error)"=w1168, "Output"=w1160, "Control Mode"=w1159, "PhoenixMotorControlDevRef"=w1167) -> ("error out"=w1152:errorcluster, "PhoenixMotorControlDevRef"=w1151:T9)  [unwired: 6 in]
        n252 = call <vilib>:"CTRE_Phoenix_MotorControl_Set.vi"("error in (no error)"=w1148, "Output"=-0.55, "Control Mode"=w1146, "PhoenixMotorControlDevRef"=w1147) -> ("error out"=w1144:errorcluster, "PhoenixMotorControlDevRef"=w1143:T9)  [unwired: 6 in]
        n253 = call "Drive_Vi.vi"("Middle Thumb"=w1156, "Z"=w1155, "Y"=w1154, "X"=w1153) -> ()  [unwired: 8 in]
      }
      n254 = while {
        tunnel: w841 -> [w922]
        tunnel: w840 -> [w921]
        i -> [w914]
        stop <- w913 stop-if-true
        n255 = for {
          N: 20 -> [_]
          tunnel: w922 -> [w934]
          tunnel: w921 -> [w933]
          tunnel: [w932] -> w920 mode=indexing
          tunnel: [w931] -> w919 mode=indexing
          w929 = T13 0 items=["PercentOutput"=0, "Position"=1, "Velocity"=2, "Current"=3, "Follower"=5, "MotionProfile"=6, "MotionMagic"=7, "MotionProfileArc"=10, "Disabled"=15] ("Control Mode")
          n256 = call <vilib>:"CTRE_Phoenix_MotorControl_Set.vi"("error in (no error)"=w933, "Output"=-0.1, "Control Mode"=w929, "PhoenixMotorControlDevRef"=w934) -> ("error out"=w931:errorcluster, "PhoenixMotorControlDevRef"=w932:T9)  [unwired: 6 in]
          n257 = Wait (ms)(milliseconds to wait=u32 35) -> ()  [unwired: 1 out]
        }
        n258 = for {
          N: 20 -> [_]
          tunnel: w920 -> [w927] mode=indexing
          tunnel: w919 -> [w926] mode=indexing
          w924 = T13 0 items=["PercentOutput"=0, "Position"=1, "Velocity"=2, "Current"=3, "Follower"=5, "MotionProfile"=6, "MotionMagic"=7, "MotionProfileArc"=10, "Disabled"=15] ("Control Mode")
          n259 = Wait (ms)(milliseconds to wait=u32 50) -> ()  [unwired: 1 out]
          n260 = call <vilib>:"CTRE_Phoenix_MotorControl_Set.vi"("error in (no error)"=w926, "Output"=0.0, "Control Mode"=w924, "PhoenixMotorControlDevRef"=w927) -> ()  [unwired: 6 in, 2 out]
        }
        n261 = Greater?(x=w914, y=2) -> (0:w913:bool)
        n262 = Wait (ms)(milliseconds to wait=u32 20) -> ()  [unwired: 1 out]
      }
      n263 = call <vilib>:"WPI_SwitchRefNum Registry Get.vi"("refnum name"="Orange Limit Switch") -> ("error out"=w880:errorcluster, "SwitchDevRef"=w879:T4)  [unwired: 9 in]
      n264 = call <vilib>:"WPI_SwitchRefNum Registry Get.vi"("refnum name"="Blue Limit Switch") -> ("error out"=w882:errorcluster, "SwitchDevRef"=w881:T4)  [unwired: 9 in]
      n265 = while {
        tunnel: w872 -> [_]
        tunnel: w871 -> [_]
        tunnel: w882 -> [w1140]
        tunnel: w881 -> [w1139]
        tunnel: w880 -> [w1138]
        tunnel: w879 -> [w1137]
        tunnel: w878 -> [w1116]
        tunnel: w877 -> [w1115]
        tunnel: w876 -> [w1111]
        tunnel: w875 -> [w1112]
        tunnel: [w1120] -> w870
        tunnel: [w1119] -> w869
        tunnel: [w1118] -> w868
        tunnel: [w1117] -> w867
        tunnel: [w1116] -> w866
        tunnel: [w1115] -> w865
        tunnel: [w1114] -> w864
        tunnel: [w1113] -> w863
        i -> [w1126]
        stop <- w1125 stop-if-true
        w1110 = T13 0 items=["PercentOutput"=0, "Position"=1, "Velocity"=2, "Current"=3, "Follower"=5, "MotionProfile"=6, "MotionMagic"=7, "MotionProfileArc"=10, "Disabled"=15] ("Control Mode")
        n266 = call <vilib>:"WPI_SwitchGetLimitValue.vi"("error in (no error)"=w1138, "SwitchDevRef"=w1137) -> ("error out"=w1117:errorcluster, "Switch Pressed"=w1136:bool, "SwitchDevRef"=w1118:T4)  [unwired: 7 in]
        "Orange Limit Pressed 3" <- w1136
        n267 = call <vilib>:"WPI_SwitchGetLimitValue.vi"("error in (no error)"=w1140, "SwitchDevRef"=w1139) -> ("error out"=w1119:errorcluster, "Switch Pressed"=w1135:bool, "SwitchDevRef"=w1120:T4)  [unwired: 7 in]
        "Blue Limit Pressed 3" <- w1135
        n268 = call-poly <vilib>:"NT Read Value.vi"("Default Value"=0.0, "Name"="/limelight-drtrain/ty") -> ("Numeric"=w1130:dbl)  [unwired: 8 in, 1 out]
        "Ty 3" <- w1130
        n269 = Greater?(x=w1126, y=5) -> (0:w1125:bool)
        n270 = call "Turret_Aim.vi"("View Button"=FALSE ("Driver Right Thumb"), "Left Trigger"=2.0, "Orange Limit Pressed"=w1135, "Blue Limit Pressed"=w1136, "Right Bumper"=FALSE, "Left Bumper"=FALSE) -> ()  [unwired: 6 in]
        n271 = call "Shooter_Equation.vi"("Right Trigger"=2.0, "Ty"=w1130) -> ()  [unwired: 10 in]
        n272 = Wait (ms)(milliseconds to wait=u32 100) -> ()  [unwired: 1 out]
        n273 = call "Drive_Vi.vi"("Middle Thumb"=FALSE, "Z"=0.0, "Y"=0.15, "X"=0.0) -> ()  [unwired: 8 in]
        n274 = call <vilib>:"CTRE_Phoenix_MotorControl_Set.vi"("error in (no error)"=w1111, "Output"=0.0, "Control Mode"=w1110, "PhoenixMotorControlDevRef"=w1112) -> ("error out"=w1113:errorcluster, "PhoenixMotorControlDevRef"=w1114:T9)  [unwired: 6 in]
      }
      n275 = while {
        tunnel: w869 -> [w1106]
        tunnel: w870 -> [w1105]
        tunnel: w867 -> [w1104]
        tunnel: w866 -> [w1091]
        tunnel: w865 -> [w1090]
        tunnel: w863 -> [w1089]
        tunnel: w864 -> [w1088]
        tunnel: w868 -> [w1079]
        tunnel: [w1078] -> w862
        tunnel: [w1077] -> w861
        tunnel: [w1076] -> w860
        tunnel: [w1075] -> w859
        i -> [w1093]
        stop <- w1092 stop-if-true
        w1086 = T13 0 items=["PercentOutput"=0, "Position"=1, "Velocity"=2, "Current"=3, "Follower"=5, "MotionProfile"=6, "MotionMagic"=7, "MotionProfileArc"=10, "Disabled"=15] ("Control Mode")
        w1087 = T13 0 items=["PercentOutput"=0, "Position"=1, "Velocity"=2, "Current"=3, "Follower"=5, "MotionProfile"=6, "MotionMagic"=7, "MotionProfileArc"=10, "Disabled"=15] ("Control Mode")
        # "40"
        n276 = call <vilib>:"WPI_SwitchGetLimitValue.vi"("error in (no error)"=w1104, "SwitchDevRef"=w1079) -> ("Switch Pressed"=w1103:bool)  [unwired: 7 in, 2 out]
        "Orange Limit Pressed 4" <- w1103
        n277 = call <vilib>:"WPI_SwitchGetLimitValue.vi"("error in (no error)"=w1106, "SwitchDevRef"=w1105) -> ("Switch Pressed"=w1102:bool)  [unwired: 7 in, 2 out]
        "Blue Limit Pressed 4" <- w1102
        n278 = call-poly <vilib>:"NT Read Value.vi"("Default Value"=0.0, "Name"="/limelight-drtrain/ty") -> ("Numeric"=w1097:dbl)  [unwired: 8 in, 1 out]
        "Ty 4" <- w1097
        n279 = Greater?(x=w1093, y=20) -> (0:w1092:bool)
        n280 = call "Turret_Aim.vi"("View Button"=FALSE ("Driver Right Thumb"), "Left Trigger"=2.0, "Orange Limit Pressed"=w1102, "Blue Limit Pressed"=w1103, "Right Bumper"=FALSE, "Left Bumper"=FALSE) -> ()  [unwired: 6 in]
        n281 = call "Shooter_Equation.vi"("Right Trigger"=2.0, "Ty"=w1097) -> ()  [unwired: 10 in]
        n282 = Wait (ms)(milliseconds to wait=u32 100) -> ()  [unwired: 1 out]
        n283 = call "Drive_Vi.vi"("Middle Thumb"=FALSE, "Z"=0.0, "Y"=0.15, "X"=0.0) -> ()  [unwired: 8 in]
        n284 = call <vilib>:"CTRE_Phoenix_MotorControl_Set.vi"("error in (no error)"=w1089, "Output"=0.35, "Control Mode"=w1086, "PhoenixMotorControlDevRef"=w1088) -> ("error out"=w1078:errorcluster, "PhoenixMotorControlDevRef"=w1077:T9)  [unwired: 6 in]
        n285 = call <vilib>:"CTRE_Phoenix_MotorControl_Set.vi"("error in (no error)"=w1091, "Output"=-0.35, "Control Mode"=w1087, "PhoenixMotorControlDevRef"=w1090) -> ("error out"=w1075:errorcluster, "PhoenixMotorControlDevRef"=w1076:T9)  [unwired: 6 in]
      }
      n286 = while {
        tunnel: w862 -> [w1070]
        tunnel: w861 -> [w1069]
        tunnel: w860 -> [w1068]
        tunnel: w859 -> [w1067]
        tunnel: [w1058] -> w839
        tunnel: [w1057] -> w837
        tunnel: [w1056] -> w835
        tunnel: [w1055] -> w833
        i -> [w1065]
        stop <- w1064 stop-if-true
        w1073 = T13 0 items=["PercentOutput"=0, "Position"=1, "Velocity"=2, "Current"=3, "Follower"=5, "MotionProfile"=6, "MotionMagic"=7, "MotionProfileArc"=10, "Disabled"=15] ("Control Mode")
        w1074 = T13 0 items=["PercentOutput"=0, "Position"=1, "Velocity"=2, "Current"=3, "Follower"=5, "MotionProfile"=6, "MotionMagic"=7, "MotionProfileArc"=10, "Disabled"=15] ("Control Mode")
        n287 = call <vilib>:"CTRE_Phoenix_MotorControl_Set.vi"("error in (no error)"=w1070, "Output"=0.0, "Control Mode"=w1073, "PhoenixMotorControlDevRef"=w1069) -> ("error out"=w1057:errorcluster, "PhoenixMotorControlDevRef"=w1058:T9)  [unwired: 6 in]
        n288 = call <vilib>:"CTRE_Phoenix_MotorControl_Set.vi"("error in (no error)"=w1067, "Output"=0.0, "Control Mode"=w1074, "PhoenixMotorControlDevRef"=w1068) -> ("error out"=w1055:errorcluster, "PhoenixMotorControlDevRef"=w1056:T9)  [unwired: 6 in]
        n289 = call "Drive_Vi.vi"("Middle Thumb"=FALSE, "Z"=-0.35, "Y"=0.0, "X"=0.0) -> ()  [unwired: 8 in]
        n290 = Greater?(x=w1065, y=5) -> (0:w1064:bool)
        n291 = Wait (ms)(milliseconds to wait=u32 100) -> ()  [unwired: 1 out]
        n292 = call-poly <vilib>:"NT Read Value.vi"("Default Value"=0.0, "Name"="/limelight-drtrain/ty") -> ("Numeric"=w1060:dbl)  [unwired: 8 in, 1 out]
        "Ty 9" <- w1060
        n293 = call "Shooter_Equation.vi"("Right Trigger"=0.0, "Ty"=w1060) -> ()  [unwired: 10 in]
      }
      n294 = while {
        tunnel: [w904] -> w838
        tunnel: w839 -> [w904]
        tunnel: [w903] -> w836
        tunnel: w837 -> [w903]
        tunnel: [w902] -> w834
        tunnel: w835 -> [w902]
        tunnel: [w901] -> w832
        tunnel: w833 -> [w901]
        i -> [w910]
        stop <- w911 stop-if-true
        n295 = Wait (ms)(milliseconds to wait=u32 20) -> ()  [unwired: 1 out]
        n296 = Greater?(x=w910, y=5) -> (0:w911:bool)
        n297 = call "Drive_Vi.vi"("Middle Thumb"=TRUE, "Z"=0.0, "Y"=0.0, "X"=0.0) -> ()  [unwired: 8 in]
      }
      n298 = while {
        tunnel: w838 -> [w1034]
        tunnel: w836 -> [w1033]
        tunnel: w834 -> [w1032]
        tunnel: w832 -> [w1031]
        tunnel: [w1030] -> w858
        tunnel: [w1029] -> w857
        tunnel: [w1028] -> w856
        tunnel: [w1027] -> w855
        i -> [w1045]
        stop <- w1044 stop-if-true
        w1049 = T13 0 items=["PercentOutput"=0, "Position"=1, "Velocity"=2, "Current"=3, "Follower"=5, "MotionProfile"=6, "MotionMagic"=7, "MotionProfileArc"=10, "Disabled"=15] ("Control Mode")
        w1050 = T13 0 items=["PercentOutput"=0, "Position"=1, "Velocity"=2, "Current"=3, "Follower"=5, "MotionProfile"=6, "MotionMagic"=7, "MotionProfileArc"=10, "Disabled"=15] ("Control Mode")
        # "-0.186"
        # "-0.944"
        # ".135"
        n299 = call "Drive_Vi.vi"("Middle Thumb"=FALSE, "Z"=0.0, "Y"=-0.8, "X"=0.0) -> ()  [unwired: 8 in]
        n300 = call <vilib>:"CTRE_Phoenix_MotorControl_Set.vi"("error in (no error)"=w1033, "Output"=0.0, "Control Mode"=w1049, "PhoenixMotorControlDevRef"=w1034) -> ("error out"=w1029:errorcluster, "PhoenixMotorControlDevRef"=w1030:T9)  [unwired: 6 in]
        n301 = call <vilib>:"CTRE_Phoenix_MotorControl_Set.vi"("error in (no error)"=w1031, "Output"=0.0, "Control Mode"=w1050, "PhoenixMotorControlDevRef"=w1032) -> ("error out"=w1027:errorcluster, "PhoenixMotorControlDevRef"=w1028:T9)  [unwired: 6 in]
        n302 = Greater?(x=w1045, y=8) -> (0:w1044:bool)
        n303 = Wait (ms)(milliseconds to wait=u32 100) -> ()  [unwired: 1 out]
        n304 = call-poly <vilib>:"NT Read Value.vi"("Default Value"=0.0, "Name"="/limelight-drtrain/ty") -> ("Numeric"=w1036:dbl)  [unwired: 8 in, 1 out]
        "Ty 10" <- w1036
        n305 = call "Shooter_Equation.vi"("Right Trigger"=0.0, "Ty"=w1036) -> ()  [unwired: 10 in]
      }
      n306 = while {
        tunnel: w858 -> [w1018]
        tunnel: w857 -> [w1017]
        tunnel: w856 -> [w1016]
        tunnel: w855 -> [w1015]
        tunnel: [w1010] -> w854
        tunnel: [w1009] -> w853
        tunnel: [w1008] -> w852
        tunnel: [w1007] -> w851
        i -> [w1012]
        stop <- w1011 stop-if-true
        w1025 = T13 0 items=["PercentOutput"=0, "Position"=1, "Velocity"=2, "Current"=3, "Follower"=5, "MotionProfile"=6, "MotionMagic"=7, "MotionProfileArc"=10, "Disabled"=15] ("Control Mode")
        w1026 = T13 0 items=["PercentOutput"=0, "Position"=1, "Velocity"=2, "Current"=3, "Follower"=5, "MotionProfile"=6, "MotionMagic"=7, "MotionProfileArc"=10, "Disabled"=15] ("Control Mode")
        # "-0.186"
        # "-0.944"
        # ".135"
        n307 = call <vilib>:"CTRE_Phoenix_MotorControl_Set.vi"("error in (no error)"=w1017, "Output"=0.0, "Control Mode"=w1025, "PhoenixMotorControlDevRef"=w1018) -> ("error out"=w1009:errorcluster, "PhoenixMotorControlDevRef"=w1010:T9)  [unwired: 6 in]
        n308 = call <vilib>:"CTRE_Phoenix_MotorControl_Set.vi"("error in (no error)"=w1015, "Output"=0.0, "Control Mode"=w1026, "PhoenixMotorControlDevRef"=w1016) -> ("error out"=w1007:errorcluster, "PhoenixMotorControlDevRef"=w1008:T9)  [unwired: 6 in]
        n309 = call "Drive_Vi.vi"("Middle Thumb"=FALSE, "Z"=0.0, "Y"=0.0, "X"=0.0) -> ()  [unwired: 8 in]
        n310 = Greater?(x=w1012, y=5) -> (0:w1011:bool)
        n311 = call-poly <vilib>:"NT Read Value.vi"("Default Value"=0.0, "Name"="/limelight-drtrain/ty") -> ("Numeric"=w1020:dbl)  [unwired: 8 in, 1 out]
        "Ty 11" <- w1020
        n312 = Wait (ms)(milliseconds to wait=u32 100) -> ()  [unwired: 1 out]
        n313 = call "Shooter_Equation.vi"("Right Trigger"=0.0, "Ty"=w1020) -> ()  [unwired: 10 in]
      }
      n314 = while {
        tunnel: w854 -> [w990]
        tunnel: w853 -> [w989]
        tunnel: w852 -> [w988]
        tunnel: w851 -> [w987]
        tunnel: [w982] -> w850
        tunnel: [w981] -> w849
        tunnel: [w980] -> w848
        tunnel: [w979] -> w847
        i -> [w984]
        stop <- w983 stop-if-true
        w1001 = T13 0 items=["PercentOutput"=0, "Position"=1, "Velocity"=2, "Current"=3, "Follower"=5, "MotionProfile"=6, "MotionMagic"=7, "MotionProfileArc"=10, "Disabled"=15] ("Control Mode")
        w1002 = T13 0 items=["PercentOutput"=0, "Position"=1, "Velocity"=2, "Current"=3, "Follower"=5, "MotionProfile"=6, "MotionMagic"=7, "MotionProfileArc"=10, "Disabled"=15] ("Control Mode")
        # "-0.186"
        # "-0.944"
        # ".135"
        n315 = call "Drive_Vi.vi"("Middle Thumb"=FALSE, "Z"=0.0, "Y"=0.0, "X"=0.0) -> ()  [unwired: 8 in]
        n316 = call <vilib>:"CTRE_Phoenix_MotorControl_Set.vi"("error in (no error)"=w989, "Output"=0.75, "Control Mode"=w1001, "PhoenixMotorControlDevRef"=w990) -> ("error out"=w981:errorcluster, "PhoenixMotorControlDevRef"=w982:T9)  [unwired: 6 in]
        n317 = call <vilib>:"CTRE_Phoenix_MotorControl_Set.vi"("error in (no error)"=w987, "Output"=-0.1, "Control Mode"=w1002, "PhoenixMotorControlDevRef"=w988) -> ("error out"=w979:errorcluster, "PhoenixMotorControlDevRef"=w980:T9)  [unwired: 6 in]
        n318 = Greater?(x=w984, y=20) -> (0:w983:bool)
        n319 = Wait (ms)(milliseconds to wait=u32 100) -> ()  [unwired: 1 out]
        n320 = call-poly <vilib>:"NT Read Value.vi"("Default Value"=0.0, "Name"="/limelight-drtrain/ty") -> ("Numeric"=w992:dbl)  [unwired: 8 in, 1 out]
        "Ty 12" <- w992
        n321 = call "Shooter_Equation.vi"("Right Trigger"=0.0, "Ty"=w992) -> ()  [unwired: 10 in]
      }
      n322 = while {
        tunnel: w850 -> [w966]
        tunnel: [w959] -> _
        tunnel: w848 -> [w965]
        tunnel: w847 -> [w964]
        tunnel: w849 -> [w959]
        tunnel: [w958] -> w846
        tunnel: [w957] -> w845
        tunnel: [w956] -> w844
        tunnel: [w955] -> w843
        i -> [w961]
        stop <- w960 stop-if-true
        w977 = T13 0 items=["PercentOutput"=0, "Position"=1, "Velocity"=2, "Current"=3, "Follower"=5, "MotionProfile"=6, "MotionMagic"=7, "MotionProfileArc"=10, "Disabled"=15] ("Control Mode")
        w978 = T13 0 items=["PercentOutput"=0, "Position"=1, "Velocity"=2, "Current"=3, "Follower"=5, "MotionProfile"=6, "MotionMagic"=7, "MotionProfileArc"=10, "Disabled"=15] ("Control Mode")
        # "-0.186"
        # "-0.944"
        # ".135"
        n323 = call "Drive_Vi.vi"("Middle Thumb"=FALSE, "Z"=0.0, "Y"=0.0, "X"=0.0) -> ()  [unwired: 8 in]
        n324 = call <vilib>:"CTRE_Phoenix_MotorControl_Set.vi"("error in (no error)"=w959, "Output"=0.0, "Control Mode"=w977, "PhoenixMotorControlDevRef"=w966) -> ("error out"=w955:errorcluster, "PhoenixMotorControlDevRef"=w956:T9)  [unwired: 6 in]
        n325 = call <vilib>:"CTRE_Phoenix_MotorControl_Set.vi"("error in (no error)"=w964, "Output"=0.0, "Control Mode"=w978, "PhoenixMotorControlDevRef"=w965) -> ("error out"=w958:errorcluster, "PhoenixMotorControlDevRef"=w957:T9)  [unwired: 6 in]
        n326 = Greater?(x=w961, y=10) -> (0:w960:bool)
        n327 = Wait (ms)(milliseconds to wait=u32 100) -> ()  [unwired: 1 out]
        n328 = call-poly <vilib>:"NT Read Value.vi"("Default Value"=0.0, "Name"="/limelight-drtrain/ty") -> ("Numeric"=w968:dbl)  [unwired: 8 in, 1 out]
        "Ty 13" <- w968
        n329 = call "Shooter_Equation.vi"("Right Trigger"=0.0, "Ty"=w968) -> ()  [unwired: 10 in]
      }
      n330 = while {
        tunnel: w844 -> [w942]
        tunnel: [w935] -> _
        tunnel: w845 -> [w941]
        tunnel: w846 -> [w940]
        tunnel: w843 -> [w935]
        i -> [w937]
        stop <- w936 stop-if-true
        w953 = T13 0 items=["PercentOutput"=0, "Position"=1, "Velocity"=2, "Current"=3, "Follower"=5, "MotionProfile"=6, "MotionMagic"=7, "MotionProfileArc"=10, "Disabled"=15] ("Control Mode")
        w954 = T13 0 items=["PercentOutput"=0, "Position"=1, "Velocity"=2, "Current"=3, "Follower"=5, "MotionProfile"=6, "MotionMagic"=7, "MotionProfileArc"=10, "Disabled"=15] ("Control Mode")
        # "-0.186"
        # "-0.944"
        # ".135"
        n331 = call "Drive_Vi.vi"("Middle Thumb"=FALSE, "Z"=0.0, "Y"=0.0, "X"=0.0) -> ()  [unwired: 8 in]
        n332 = call <vilib>:"CTRE_Phoenix_MotorControl_Set.vi"("error in (no error)"=w935, "Output"=0.0, "Control Mode"=w953, "PhoenixMotorControlDevRef"=w942) -> ()  [unwired: 6 in, 2 out]
        n333 = call <vilib>:"CTRE_Phoenix_MotorControl_Set.vi"("error in (no error)"=w940, "Output"=0.0, "Control Mode"=w954, "PhoenixMotorControlDevRef"=w941) -> ()  [unwired: 6 in, 2 out]
        n334 = Greater?(x=w937, y=20) -> (0:w936:bool)
        n335 = Wait (ms)(milliseconds to wait=u32 100) -> ()  [unwired: 1 out]
        n336 = call-poly <vilib>:"NT Read Value.vi"("Default Value"=0.0, "Name"="/limelight-drtrain/ty") -> ("Numeric"=w944:dbl)  [unwired: 8 in, 1 out]
        "Ty 14" <- w944
        n337 = call "Shooter_Equation.vi"("Right Trigger"=0.0, "Ty"=w944) -> ()  [unwired: 10 in]
      }
    }
    frame "4 Ball Pos 3" {
      # "Pigeon Set"
      n338 = while {
        i -> [w1633]
        stop <- w1634 stop-if-true
        n339 = Wait (ms)(milliseconds to wait=u32 20) -> ()  [unwired: 1 out]
        n340 = Greater?(x=w1633, y=2) -> (0:w1634:bool)
        n341 = call "Drive_Vi.vi"("Middle Thumb"=TRUE, "Z"=0.0, "Y"=0.0, "X"=0.0) -> ()  [unwired: 8 in]
      }
      n342 = call <vilib>:"WPI_SwitchRefNum Registry Get.vi"("refnum name"="Intake Sensor") -> ("error out"=w1286:errorcluster, "SwitchDevRef"=w1285:T4)  [unwired: 9 in]
      n343 = call <vilib>:"CTRE_Phoenix_MotorControl_RefNumRegistryGet.vi"("refnum name"="Intake") -> ("error out"=w1280:errorcluster, "PhoenixMotorControlDevRef"=w1279:T9)  [unwired: 9 in]
      n344 = call <vilib>:"CTRE_Phoenix_MotorControl_RefNumRegistryGet.vi"("refnum name"="Reject") -> ("error out"=w1282:errorcluster, "PhoenixMotorControlDevRef"=w1281:T9)  [unwired: 9 in]
      n345 = call "Limit_Switches.vi"() -> ()  [unwired: 10 in, 2 out]
      n346 = call <vilib>:"CTRE_Phoenix_MotorControl_RefNumRegistryGet.vi"("refnum name"="Elevate") -> ("error out"=w1284:errorcluster, "PhoenixMotorControlDevRef"=w1283:T9)  [unwired: 9 in]
      n347 = call <vilib>:"WPI_SwitchRefNum Registry Get.vi"("refnum name"="Elevate Sensor") -> ("error out"=w1288:errorcluster, "SwitchDevRef"=w1287:T4)  [unwired: 9 in]
      n348 = call <vilib>:"CTRE_Phoenix_MotorControl_RefNumRegistryGet.vi"("refnum name"="Shoot") -> ("error out"=w1268:errorcluster, "PhoenixMotorControlDevRef"=w1267:T9)  [unwired: 9 in]
      n349 = call <vilib>:"CTRE_Phoenix_MotorControl_RefNumRegistryGet.vi"("refnum name"="Intake Actuate") -> ("error out"=w1238:errorcluster, "PhoenixMotorControlDevRef"=w1239:T9)  [unwired: 9 in]
      n350 = while {
        tunnel: w1288 -> [w1592]
        tunnel: w1287 -> [w1591]
        tunnel: w1286 -> [w1590]
        tunnel: w1285 -> [w1589]
        tunnel: w1284 -> [w1586]
        tunnel: w1283 -> [w1585]
        tunnel: w1282 -> [w1584]
        tunnel: w1281 -> [w1583]
        tunnel: w1280 -> [w1582]
        tunnel: w1279 -> [w1581]
        tunnel: [w1570] -> w1272
        tunnel: [w1569] -> w1271
        tunnel: [w1568] -> w1270
        tunnel: [w1567] -> w1269
        tunnel: w1268 -> [w1566]
        tunnel: w1267 -> [w1565]
        tunnel: [w1562] -> w1266
        tunnel: [w1561] -> w1265
        i -> [w1595]
        stop <- w1596 stop-if-true
        w1564 = T13 0 items=["PercentOutput"=0, "Position"=1, "Velocity"=2, "Current"=3, "Follower"=5, "MotionProfile"=6, "MotionMagic"=7, "MotionProfileArc"=10, "Disabled"=15] ("Control Mode")
        w1575 = T13 0 items=["PercentOutput"=0, "Position"=1, "Velocity"=2, "Current"=3, "Follower"=5, "MotionProfile"=6, "MotionMagic"=7, "MotionProfileArc"=10, "Disabled"=15] ("Control Mode")
        w1576 = T13 0 items=["PercentOutput"=0, "Position"=1, "Velocity"=2, "Current"=3, "Follower"=5, "MotionProfile"=6, "MotionMagic"=7, "MotionProfileArc"=10, "Disabled"=15] ("Control Mode")
        w1577 = T13 0 items=["PercentOutput"=0, "Position"=1, "Velocity"=2, "Current"=3, "Follower"=5, "MotionProfile"=6, "MotionMagic"=7, "MotionProfileArc"=10, "Disabled"=15] ("Control Mode")
        n351 = call <vilib>:"WPI_SwitchGetLimitValue.vi"("error in (no error)"=w1590, "SwitchDevRef"=w1589) -> ("Switch Pressed"=w1593:bool)  [unwired: 7 in, 2 out]
        n352 = call <vilib>:"WPI_SwitchGetLimitValue.vi"("error in (no error)"=w1592, "SwitchDevRef"=w1591) -> ("Switch Pressed"=w1594:bool)  [unwired: 7 in, 2 out]
        n353 = Greater?(x=w1595, y=20) -> (0:w1596:bool)
        n354 = Not(x=w1593) -> (.not. x?=w1580:bool)
        "Intake 5" <- w1580
        n355 = Not(x=w1594) -> (.not. x?=w1588:bool)
        "Elevate 5" <- w1588
        n356 = Wait (ms)(milliseconds to wait=u32 100) -> ()  [unwired: 1 out]
        n357 = case shown="True" w1588 {
          tunnel: [0.75 ("Output") w1613] -> w1587
          tunnel: w1580 -> [_ w1610]
          tunnel: [0.75 ("Output") w1612] -> w1579
          tunnel: [-0.1 ("Output") w1611] -> w1578
          tunnel: [FALSE ("Middle Thumb") w1609] -> w1574
          tunnel: [0.0 ("Z") w1608] -> w1573
          tunnel: [0.0 ("Y") w1607] -> w1572
          tunnel: [0.0 ("X") w1606] -> w1571
          frame False {
            (unwired) WPI_SolenoidValue."Reverse" ("Value")
          }
          frame True {
            n358 = case shown="True" w1610 {
              tunnel: [0.75 ("Output") 0.0 ("Output")] -> w1613
              tunnel: [0.0 ("Output") 0.0 ("Output")] -> w1612
              tunnel: [0.0 ("Output") 0.0 ("Output")] -> w1611
              tunnel: [FALSE ("Middle Thumb") FALSE ("Middle Thumb")] -> w1609
              tunnel: [0.0 ("Z") 0.0 ("Z")] -> w1608
              tunnel: [-0.3 ("Y") 0.0 ("Y")] -> w1607
              tunnel: [0.0 ("X") 0.0 ("X")] -> w1606
              frame False {
              }
              frame True {
              }
            }
          }
        }
        n359 = call <vilib>:"CTRE_Phoenix_MotorControl_Set.vi"("error in (no error)"=w1582, "Output"=w1587, "Control Mode"=w1575, "PhoenixMotorControlDevRef"=w1581) -> ("error out"=w1568:errorcluster, "PhoenixMotorControlDevRef"=w1567:T9)  [unwired: 6 in]
        n360 = call <vilib>:"CTRE_Phoenix_MotorControl_Set.vi"("error in (no error)"=w1584, "Output"=w1579, "Control Mode"=w1576, "PhoenixMotorControlDevRef"=w1583) -> ()  [unwired: 6 in, 2 out]
        n361 = call <vilib>:"CTRE_Phoenix_MotorControl_Set.vi"("error in (no error)"=w1586, "Output"=w1578, "Control Mode"=w1577, "PhoenixMotorControlDevRef"=w1585) -> ("error out"=w1570:errorcluster, "PhoenixMotorControlDevRef"=w1569:T9)  [unwired: 6 in]
        n362 = call <vilib>:"CTRE_Phoenix_MotorControl_Set.vi"("error in (no error)"=w1566, "Output"=-0.55, "Control Mode"=w1564, "PhoenixMotorControlDevRef"=w1565) -> ("error out"=w1562:errorcluster, "PhoenixMotorControlDevRef"=w1561:T9)  [unwired: 6 in]
        n363 = call "Drive_Vi.vi"("Middle Thumb"=w1574, "Z"=w1573, "Y"=w1572, "X"=w1571) -> ()  [unwired: 8 in]
      }
      n364 = while {
        tunnel: w1239 -> [w1328]
        tunnel: w1238 -> [w1327]
        i -> [w1320]
        stop <- w1319 stop-if-true
        n365 = for {
          N: 20 -> [_]
          tunnel: w1328 -> [w1340]
          tunnel: w1327 -> [w1339]
          tunnel: [w1338] -> w1326 mode=indexing
          tunnel: [w1337] -> w1325 mode=indexing
          w1335 = T13 0 items=["PercentOutput"=0, "Position"=1, "Velocity"=2, "Current"=3, "Follower"=5, "MotionProfile"=6, "MotionMagic"=7, "MotionProfileArc"=10, "Disabled"=15] ("Control Mode")
          n366 = call <vilib>:"CTRE_Phoenix_MotorControl_Set.vi"("error in (no error)"=w1339, "Output"=-0.1, "Control Mode"=w1335, "PhoenixMotorControlDevRef"=w1340) -> ("error out"=w1337:errorcluster, "PhoenixMotorControlDevRef"=w1338:T9)  [unwired: 6 in]
          n367 = Wait (ms)(milliseconds to wait=u32 35) -> ()  [unwired: 1 out]
        }
        n368 = for {
          N: 20 -> [_]
          tunnel: w1326 -> [w1333] mode=indexing
          tunnel: w1325 -> [w1332] mode=indexing
          w1330 = T13 0 items=["PercentOutput"=0, "Position"=1, "Velocity"=2, "Current"=3, "Follower"=5, "MotionProfile"=6, "MotionMagic"=7, "MotionProfileArc"=10, "Disabled"=15] ("Control Mode")
          n369 = Wait (ms)(milliseconds to wait=u32 50) -> ()  [unwired: 1 out]
          n370 = call <vilib>:"CTRE_Phoenix_MotorControl_Set.vi"("error in (no error)"=w1332, "Output"=0.0, "Control Mode"=w1330, "PhoenixMotorControlDevRef"=w1333) -> ()  [unwired: 6 in, 2 out]
        }
        n371 = Greater?(x=w1320, y=2) -> (0:w1319:bool)
        n372 = Wait (ms)(milliseconds to wait=u32 20) -> ()  [unwired: 1 out]
      }
      n373 = call <vilib>:"WPI_SwitchRefNum Registry Get.vi"("refnum name"="Orange Limit Switch") -> ("error out"=w1274:errorcluster, "SwitchDevRef"=w1273:T4)  [unwired: 9 in]
      n374 = call <vilib>:"WPI_SwitchRefNum Registry Get.vi"("refnum name"="Blue Limit Switch") -> ("error out"=w1276:errorcluster, "SwitchDevRef"=w1275:T4)  [unwired: 9 in]
      n375 = while {
        tunnel: w1266 -> [_]
        tunnel: w1265 -> [_]
        tunnel: w1276 -> [w1558]
        tunnel: w1275 -> [w1557]
        tunnel: w1274 -> [w1556]
        tunnel: w1273 -> [w1555]
        tunnel: w1272 -> [w1534]
        tunnel: w1271 -> [w1533]
        tunnel: w1270 -> [w1529]
        tunnel: w1269 -> [w1530]
        tunnel: [w1538] -> w1264
        tunnel: [w1537] -> w1263
        tunnel: [w1536] -> w1262
        tunnel: [w1535] -> w1261
        tunnel: [w1534] -> w1260
        tunnel: [w1533] -> w1259
        tunnel: [w1532] -> w1258
        tunnel: [w1531] -> w1257
        i -> [w1544]
        stop <- w1543 stop-if-true
        w1528 = T13 0 items=["PercentOutput"=0, "Position"=1, "Velocity"=2, "Current"=3, "Follower"=5, "MotionProfile"=6, "MotionMagic"=7, "MotionProfileArc"=10, "Disabled"=15] ("Control Mode")
        n376 = call <vilib>:"WPI_SwitchGetLimitValue.vi"("error in (no error)"=w1556, "SwitchDevRef"=w1555) -> ("error out"=w1535:errorcluster, "Switch Pressed"=w1554:bool, "SwitchDevRef"=w1536:T4)  [unwired: 7 in]
        "Orange Limit Pressed 9" <- w1554
        n377 = call <vilib>:"WPI_SwitchGetLimitValue.vi"("error in (no error)"=w1558, "SwitchDevRef"=w1557) -> ("error out"=w1537:errorcluster, "Switch Pressed"=w1553:bool, "SwitchDevRef"=w1538:T4)  [unwired: 7 in]
        "Blue Limit Pressed 9" <- w1553
        n378 = call-poly <vilib>:"NT Read Value.vi"("Default Value"=0.0, "Name"="/limelight-drtrain/ty") -> ("Numeric"=w1548:dbl)  [unwired: 8 in, 1 out]
        "Ty 15" <- w1548
        n379 = Greater?(x=w1544, y=5) -> (0:w1543:bool)
        n380 = call "Turret_Aim.vi"("View Button"=FALSE ("Driver Right Thumb"), "Left Trigger"=2.0, "Orange Limit Pressed"=w1553, "Blue Limit Pressed"=w1554, "Right Bumper"=FALSE, "Left Bumper"=FALSE) -> ()  [unwired: 6 in]
        n381 = call "Shooter_Equation.vi"("Right Trigger"=2.0, "Ty"=w1548) -> ()  [unwired: 10 in]
        n382 = Wait (ms)(milliseconds to wait=u32 100) -> ()  [unwired: 1 out]
        n383 = call "Drive_Vi.vi"("Middle Thumb"=FALSE, "Z"=0.0, "Y"=0.15, "X"=0.0) -> ()  [unwired: 8 in]
        n384 = call <vilib>:"CTRE_Phoenix_MotorControl_Set.vi"("error in (no error)"=w1529, "Output"=0.0, "Control Mode"=w1528, "PhoenixMotorControlDevRef"=w1530) -> ("error out"=w1531:errorcluster, "PhoenixMotorControlDevRef"=w1532:T9)  [unwired: 6 in]
      }
      n385 = while {
        tunnel: w1263 -> [w1524]
        tunnel: w1264 -> [w1523]
        tunnel: w1261 -> [w1522]
        tunnel: w1260 -> [w1511]
        tunnel: w1259 -> [w1510]
        tunnel: w1257 -> [w1509]
        tunnel: w1258 -> [w1508]
        tunnel: w1262 -> [w1499]
        tunnel: [w1498] -> w1256
        tunnel: [w1497] -> w1255
        tunnel: [w1496] -> w1254
        tunnel: [w1495] -> w1253
        tunnel: [w1494] -> w1221
        tunnel: [w1493] -> w1220
        i -> [w1513]
        stop <- w1512 stop-if-true
        w1506 = T13 0 items=["PercentOutput"=0, "Position"=1, "Velocity"=2, "Current"=3, "Follower"=5, "MotionProfile"=6, "MotionMagic"=7, "MotionProfileArc"=10, "Disabled"=15] ("Control Mode")
        w1507 = T13 0 items=["PercentOutput"=0, "Position"=1, "Velocity"=2, "Current"=3, "Follower"=5, "MotionProfile"=6, "MotionMagic"=7, "MotionProfileArc"=10, "Disabled"=15] ("Control Mode")
        # "40"
        n386 = call <vilib>:"WPI_SwitchGetLimitValue.vi"("error in (no error)"=w1522, "SwitchDevRef"=w1499) -> ("Switch Pressed"=w1494:bool)  [unwired: 7 in, 2 out]
        "Orange Limit Pressed 10" <- w1494
        n387 = call <vilib>:"WPI_SwitchGetLimitValue.vi"("error in (no error)"=w1524, "SwitchDevRef"=w1523) -> ("Switch Pressed"=w1493:bool)  [unwired: 7 in, 2 out]
        "Blue Limit Pressed 10" <- w1493
        n388 = call-poly <vilib>:"NT Read Value.vi"("Default Value"=0.0, "Name"="/limelight-drtrain/ty") -> ("Numeric"=w1517:dbl)  [unwired: 8 in, 1 out]
        "Ty 16" <- w1517
        n389 = Greater?(x=w1513, y=20) -> (0:w1512:bool)
        n390 = call "Turret_Aim.vi"("View Button"=FALSE ("Driver Right Thumb"), "Left Trigger"=2.0, "Orange Limit Pressed"=w1493, "Blue Limit Pressed"=w1494, "Right Bumper"=FALSE, "Left Bumper"=FALSE) -> ()  [unwired: 6 in]
        n391 = call "Shooter_Equation.vi"("Right Trigger"=2.0, "Ty"=w1517) -> ()  [unwired: 10 in]
        n392 = Wait (ms)(milliseconds to wait=u32 100) -> ()  [unwired: 1 out]
        n393 = call "Drive_Vi.vi"("Middle Thumb"=FALSE, "Z"=0.0, "Y"=0.15, "X"=0.0) -> ()  [unwired: 8 in]
        n394 = call <vilib>:"CTRE_Phoenix_MotorControl_Set.vi"("error in (no error)"=w1509, "Output"=0.35, "Control Mode"=w1506, "PhoenixMotorControlDevRef"=w1508) -> ("error out"=w1498:errorcluster, "PhoenixMotorControlDevRef"=w1497:T9)  [unwired: 6 in]
        n395 = call <vilib>:"CTRE_Phoenix_MotorControl_Set.vi"("error in (no error)"=w1511, "Output"=-0.35, "Control Mode"=w1507, "PhoenixMotorControlDevRef"=w1510) -> ("error out"=w1495:errorcluster, "PhoenixMotorControlDevRef"=w1496:T9)  [unwired: 6 in]
      }
      n396 = while {
        tunnel: w1256 -> [w1488]
        tunnel: w1255 -> [w1487]
        tunnel: w1254 -> [w1486]
        tunnel: w1253 -> [w1485]
        tunnel: [w1476] -> w1237
        tunnel: [w1475] -> w1235
        tunnel: [w1474] -> w1233
        tunnel: [w1473] -> w1231
        i -> [w1483]
        stop <- w1482 stop-if-true
        w1491 = T13 0 items=["PercentOutput"=0, "Position"=1, "Velocity"=2, "Current"=3, "Follower"=5, "MotionProfile"=6, "MotionMagic"=7, "MotionProfileArc"=10, "Disabled"=15] ("Control Mode")
        w1492 = T13 0 items=["PercentOutput"=0, "Position"=1, "Velocity"=2, "Current"=3, "Follower"=5, "MotionProfile"=6, "MotionMagic"=7, "MotionProfileArc"=10, "Disabled"=15] ("Control Mode")
        n397 = call <vilib>:"CTRE_Phoenix_MotorControl_Set.vi"("error in (no error)"=w1488, "Output"=0.0, "Control Mode"=w1491, "PhoenixMotorControlDevRef"=w1487) -> ("error out"=w1475:errorcluster, "PhoenixMotorControlDevRef"=w1476:T9)  [unwired: 6 in]
        n398 = call <vilib>:"CTRE_Phoenix_MotorControl_Set.vi"("error in (no error)"=w1485, "Output"=0.0, "Control Mode"=w1492, "PhoenixMotorControlDevRef"=w1486) -> ("error out"=w1473:errorcluster, "PhoenixMotorControlDevRef"=w1474:T9)  [unwired: 6 in]
        n399 = call "Drive_Vi.vi"("Middle Thumb"=FALSE, "Z"=0.22, "Y"=0.0, "X"=0.0) -> ()  [unwired: 8 in]
        n400 = Greater?(x=w1483, y=4) -> (0:w1482:bool)
        n401 = Wait (ms)(milliseconds to wait=u32 100) -> ()  [unwired: 1 out]
        n402 = call-poly <vilib>:"NT Read Value.vi"("Default Value"=0.0, "Name"="/limelight-drtrain/ty") -> ("Numeric"=w1478:dbl)  [unwired: 8 in, 1 out]
        "Ty 17" <- w1478
        n403 = call "Shooter_Equation.vi"("Right Trigger"=0.0, "Ty"=w1478) -> ()  [unwired: 10 in]
      }
      n404 = while {
        tunnel: [w1310] -> w1236
        tunnel: w1237 -> [w1310]
        tunnel: [w1309] -> w1234
        tunnel: w1235 -> [w1309]
        tunnel: [w1308] -> w1232
        tunnel: w1233 -> [w1308]
        tunnel: [w1307] -> w1230
        tunnel: w1231 -> [w1307]
        i -> [w1316]
        stop <- w1317 stop-if-true
        n405 = Wait (ms)(milliseconds to wait=u32 20) -> ()  [unwired: 1 out]
        n406 = Greater?(x=w1316, y=5) -> (0:w1317:bool)
        n407 = call "Drive_Vi.vi"("Middle Thumb"=TRUE, "Z"=0.0, "Y"=0.0, "X"=0.0) -> ()  [unwired: 8 in]
      }
      n408 = while {
        tunnel: w1236 -> [w1452]
        tunnel: w1234 -> [w1451]
        tunnel: w1232 -> [w1450]
        tunnel: w1230 -> [w1449]
        tunnel: [w1448] -> w1252
        tunnel: [w1447] -> w1251
        tunnel: [w1446] -> w1250
        tunnel: [w1445] -> w1249
        i -> [w1463]
        stop <- w1462 stop-if-true
        w1467 = T13 0 items=["PercentOutput"=0, "Position"=1, "Velocity"=2, "Current"=3, "Follower"=5, "MotionProfile"=6, "MotionMagic"=7, "MotionProfileArc"=10, "Disabled"=15] ("Control Mode")
        w1468 = T13 0 items=["PercentOutput"=0, "Position"=1, "Velocity"=2, "Current"=3, "Follower"=5, "MotionProfile"=6, "MotionMagic"=7, "MotionProfileArc"=10, "Disabled"=15] ("Control Mode")
        # "-0.186"
        # "-0.944"
        # ".135"
        n409 = call "Drive_Vi.vi"("Middle Thumb"=FALSE, "Z"=0.0, "Y"=-0.75, "X"=0.0) -> ()  [unwired: 8 in]
        n410 = call <vilib>:"CTRE_Phoenix_MotorControl_Set.vi"("error in (no error)"=w1451, "Output"=1.0, "Control Mode"=w1467, "PhoenixMotorControlDevRef"=w1452) -> ("error out"=w1447:errorcluster, "PhoenixMotorControlDevRef"=w1448:T9)  [unwired: 6 in]
        n411 = call <vilib>:"CTRE_Phoenix_MotorControl_Set.vi"("error in (no error)"=w1449, "Output"=0.0, "Control Mode"=w1468, "PhoenixMotorControlDevRef"=w1450) -> ("error out"=w1445:errorcluster, "PhoenixMotorControlDevRef"=w1446:T9)  [unwired: 6 in]
        n412 = Greater?(x=w1463, y=3) -> (0:w1462:bool)
        n413 = Wait (ms)(milliseconds to wait=u32 116) -> ()  [unwired: 1 out]
        n414 = call-poly <vilib>:"NT Read Value.vi"("Default Value"=0.0, "Name"="/limelight-drtrain/ty") -> ("Numeric"=w1454:dbl)  [unwired: 8 in, 1 out]
        "Ty 18" <- w1454
        n415 = call "Shooter_Equation.vi"("Right Trigger"=0.0, "Ty"=w1454) -> ()  [unwired: 10 in]
      }
      n416 = while {
        tunnel: w1252 -> [w1436]
        tunnel: w1251 -> [w1435]
        tunnel: w1250 -> [w1434]
        tunnel: w1249 -> [w1433]
        tunnel: [w1428] -> w1248
        tunnel: [w1427] -> w1247
        tunnel: [w1426] -> w1246
        tunnel: [w1425] -> w1245
        i -> [w1430]
        stop <- w1429 stop-if-true
        w1443 = T13 0 items=["PercentOutput"=0, "Position"=1, "Velocity"=2, "Current"=3, "Follower"=5, "MotionProfile"=6, "MotionMagic"=7, "MotionProfileArc"=10, "Disabled"=15] ("Control Mode")
        w1444 = T13 0 items=["PercentOutput"=0, "Position"=1, "Velocity"=2, "Current"=3, "Follower"=5, "MotionProfile"=6, "MotionMagic"=7, "MotionProfileArc"=10, "Disabled"=15] ("Control Mode")
        # "-0.186"
        # "-0.944"
        # ".135"
        n417 = call <vilib>:"CTRE_Phoenix_MotorControl_Set.vi"("error in (no error)"=w1435, "Output"=1.0, "Control Mode"=w1443, "PhoenixMotorControlDevRef"=w1436) -> ("error out"=w1427:errorcluster, "PhoenixMotorControlDevRef"=w1428:T9)  [unwired: 6 in]
        n418 = call <vilib>:"CTRE_Phoenix_MotorControl_Set.vi"("error in (no error)"=w1433, "Output"=0.0, "Control Mode"=w1444, "PhoenixMotorControlDevRef"=w1434) -> ("error out"=w1425:errorcluster, "PhoenixMotorControlDevRef"=w1426:T9)  [unwired: 6 in]
        n419 = call "Drive_Vi.vi"("Middle Thumb"=FALSE, "Z"=0.0, "Y"=0.0, "X"=0.0) -> ()  [unwired: 8 in]
        n420 = Greater?(x=w1430, y=35) -> (0:w1429:bool)
        n421 = call-poly <vilib>:"NT Read Value.vi"("Default Value"=0.0, "Name"="/limelight-drtrain/ty") -> ("Numeric"=w1438:dbl)  [unwired: 8 in, 1 out]
        "Ty 19" <- w1438
        n422 = Wait (ms)(milliseconds to wait=u32 100) -> ()  [unwired: 1 out]
        n423 = call "Shooter_Equation.vi"("Right Trigger"=0.0, "Ty"=w1438) -> ()  [unwired: 10 in]
      }
      n424 = while {
        tunnel: w1248 -> [w1408]
        tunnel: w1247 -> [w1407]
        tunnel: w1246 -> [w1406]
        tunnel: w1245 -> [w1405]
        tunnel: [w1400] -> w1244
        tunnel: [w1399] -> w1243
        tunnel: [w1398] -> w1242
        tunnel: [w1397] -> w1241
        tunnel: w1221 -> [w1391]
        tunnel: w1220 -> [w1392]
        tunnel: [w1392] -> w1219
        tunnel: [w1391] -> w1218
        i -> [w1402]
        stop <- w1401 stop-if-true
        w1419 = T13 0 items=["PercentOutput"=0, "Position"=1, "Velocity"=2, "Current"=3, "Follower"=5, "MotionProfile"=6, "MotionMagic"=7, "MotionProfileArc"=10, "Disabled"=15] ("Control Mode")
        w1420 = T13 0 items=["PercentOutput"=0, "Position"=1, "Velocity"=2, "Current"=3, "Follower"=5, "MotionProfile"=6, "MotionMagic"=7, "MotionProfileArc"=10, "Disabled"=15] ("Control Mode")
        # "-0.186"
        # "-0.944"
        # ".135"
        n425 = call "Turret_Aim.vi"("View Button"=FALSE, "Left Trigger"=0.0, "Orange Limit Pressed"=w1391, "Blue Limit Pressed"=w1392, "Right Bumper"=FALSE, "Left Bumper"=FALSE) -> ()  [unwired: 6 in]
        n426 = call "Drive_Vi.vi"("Middle Thumb"=FALSE, "Z"=0.0, "Y"=0.75, "X"=0.0) -> ()  [unwired: 8 in]
        n427 = call <vilib>:"CTRE_Phoenix_MotorControl_Set.vi"("error in (no error)"=w1407, "Output"=1.0, "Control Mode"=w1419, "PhoenixMotorControlDevRef"=w1408) -> ("error out"=w1399:errorcluster, "PhoenixMotorControlDevRef"=w1400:T9)  [unwired: 6 in]
        n428 = call <vilib>:"CTRE_Phoenix_MotorControl_Set.vi"("error in (no error)"=w1405, "Output"=-0.1, "Control Mode"=w1420, "PhoenixMotorControlDevRef"=w1406) -> ("error out"=w1397:errorcluster, "PhoenixMotorControlDevRef"=w1398:T9)  [unwired: 6 in]
        n429 = Greater?(x=w1402, y=5) -> (0:w1401:bool)
        n430 = Wait (ms)(milliseconds to wait=u32 50) -> ()  [unwired: 1 out]
        n431 = call-poly <vilib>:"NT Read Value.vi"("Default Value"=0.0, "Name"="/limelight-drtrain/ty") -> ("Numeric"=w1410:dbl)  [unwired: 8 in, 1 out]
        "Ty 20" <- w1410
        n432 = call "Shooter_Equation.vi"("Right Trigger"=0.0, "Ty"=w1410) -> ()  [unwired: 10 in]
      }
      n433 = while {
        tunnel: w1244 -> [w1378]
        tunnel: [w1371] -> _
        tunnel: w1242 -> [w1377]
        tunnel: w1241 -> [w1376]
        tunnel: w1243 -> [w1371]
        tunnel: [w1370] -> w1224
        tunnel: [w1369] -> w1223
        tunnel: [w1368] -> w1229
        tunnel: [w1367] -> w1227
        tunnel: w1219 -> [w1363]
        tunnel: w1218 -> [w1362]
        i -> [w1373]
        stop <- w1372 stop-if-true
        (unwired) FALSE ("Orange Limit Pressed")
        w1389 = T13 0 items=["PercentOutput"=0, "Position"=1, "Velocity"=2, "Current"=3, "Follower"=5, "MotionProfile"=6, "MotionMagic"=7, "MotionProfileArc"=10, "Disabled"=15] ("Control Mode")
        w1390 = T13 0 items=["PercentOutput"=0, "Position"=1, "Velocity"=2, "Current"=3, "Follower"=5, "MotionProfile"=6, "MotionMagic"=7, "MotionProfileArc"=10, "Disabled"=15] ("Control Mode")
        # "-0.186"
        # "-0.944"
        # ".135"
        n434 = call "Turret_Aim.vi"("View Button"=FALSE, "Left Trigger"=2.0, "Orange Limit Pressed"=w1362, "Blue Limit Pressed"=w1363, "Right Bumper"=FALSE, "Left Bumper"=FALSE) -> ()  [unwired: 6 in]
        n435 = call "Drive_Vi.vi"("Middle Thumb"=FALSE, "Z"=0.0, "Y"=-0.1, "X"=0.0) -> ()  [unwired: 8 in]
        n436 = call <vilib>:"CTRE_Phoenix_MotorControl_Set.vi"("error in (no error)"=w1371, "Output"=0.0, "Control Mode"=w1389, "PhoenixMotorControlDevRef"=w1378) -> ("error out"=w1367:errorcluster, "PhoenixMotorControlDevRef"=w1368:T9)  [unwired: 6 in]
        n437 = call <vilib>:"CTRE_Phoenix_MotorControl_Set.vi"("error in (no error)"=w1376, "Output"=-0.35, "Control Mode"=w1390, "PhoenixMotorControlDevRef"=w1377) -> ("error out"=w1370:errorcluster, "PhoenixMotorControlDevRef"=w1369:T9)  [unwired: 6 in]
        n438 = Greater?(x=w1373, y=10) -> (0:w1372:bool)
        n439 = Wait (ms)(milliseconds to wait=u32 100) -> ()  [unwired: 1 out]
        n440 = call-poly <vilib>:"NT Read Value.vi"("Default Value"=0.0, "Name"="/limelight-drtrain/ty") -> ("Numeric"=w1380:dbl)  [unwired: 8 in, 1 out]
        "Ty 21" <- w1380
        n441 = call "Shooter_Equation.vi"("Right Trigger"=2.0, "Ty"=w1380) -> ()  [unwired: 10 in]
      }
      n442 = while {
        tunnel: [w1306] -> w1228
        tunnel: w1229 -> [w1306]
        tunnel: [w1305] -> w1226
        tunnel: w1227 -> [w1305]
        tunnel: [w1304] -> w1225
        tunnel: w1224 -> [w1304]
        tunnel: [w1303] -> w1222
        tunnel: w1223 -> [w1303]
        i -> [w1296]
        stop <- w1295 stop-if-true
        n443 = Greater?(x=w1296, y=4) -> (0:w1295:bool)
        n444 = call "Drive_Vi.vi"("Middle Thumb"=TRUE, "Z"=0.15, "Y"=0.0, "X"=0.0) -> ()  [unwired: 8 in]
        n445 = Wait (ms)(milliseconds to wait=u32 100) -> ()  [unwired: 1 out]
      }
      n446 = while {
        tunnel: w1228 -> [w1348]
        tunnel: w1226 -> [w1341]
        tunnel: w1222 -> [w1347]
        tunnel: w1225 -> [w1346]
        i -> [w1343]
        stop <- w1342 stop-if-true
        w1359 = T13 0 items=["PercentOutput"=0, "Position"=1, "Velocity"=2, "Current"=3, "Follower"=5, "MotionProfile"=6, "MotionMagic"=7, "MotionProfileArc"=10, "Disabled"=15] ("Control Mode")
        w1360 = T13 0 items=["PercentOutput"=0, "Position"=1, "Velocity"=2, "Current"=3, "Follower"=5, "MotionProfile"=6, "MotionMagic"=7, "MotionProfileArc"=10, "Disabled"=15] ("Control Mode")
        # "-0.186"
        # "-0.944"
        # ".135"
        n447 = call "Drive_Vi.vi"("Middle Thumb"=FALSE, "Z"=0.0, "Y"=0.0, "X"=0.0) -> ()  [unwired: 8 in]
        n448 = call <vilib>:"CTRE_Phoenix_MotorControl_Set.vi"("error in (no error)"=w1341, "Output"=0.0, "Control Mode"=w1359, "PhoenixMotorControlDevRef"=w1348) -> ()  [unwired: 6 in, 2 out]
        n449 = call <vilib>:"CTRE_Phoenix_MotorControl_Set.vi"("error in (no error)"=w1346, "Output"=0.0, "Control Mode"=w1360, "PhoenixMotorControlDevRef"=w1347) -> ()  [unwired: 6 in, 2 out]
        n450 = Greater?(x=w1343, y=20) -> (0:w1342:bool)
        n451 = Wait (ms)(milliseconds to wait=u32 100) -> ()  [unwired: 1 out]
        n452 = call-poly <vilib>:"NT Read Value.vi"("Default Value"=0.0, "Name"="/limelight-drtrain/ty") -> ("Numeric"=w1350:dbl)  [unwired: 8 in, 1 out]
        "Ty 22" <- w1350
        n453 = call "Shooter_Equation.vi"("Right Trigger"=0.0, "Ty"=w1350) -> ()  [unwired: 10 in]
      }
    }
    frame "Angle Test" {
      n454 = call <vilib>:"CTRE_Phoenix_MotorControl_RefNumRegistryGet.vi"("refnum name"="Orange Back Turn") -> ("error out"=w1648:errorcluster, "PhoenixMotorControlDevRef"=w1649:T9)  [unwired: 9 in]
      n455 = call <vilib>:"CTRE_Phoenix_MotorControl_RefNumRegistryGet.vi"("refnum name"="Orange Back Drive") -> ("error out"=w1646:errorcluster, "PhoenixMotorControlDevRef"=w1647:T9)  [unwired: 9 in]
      n456 = while {
        tunnel: w1649 -> [w1692]
        tunnel: w1648 -> [w1690]
        tunnel: w1647 -> [w1685]
        tunnel: w1646 -> [w1684]
        tunnel: [w1681] -> w1643
        tunnel: [w1680] -> w1642
        tunnel: [w1679] -> w1641
        tunnel: [w1678] -> w1640
        i -> [w1695]
        stop <- w1693 stop-if-true
        w1682 = T13 0 items=["PercentOutput"=0, "Position"=1, "Velocity"=2, "Current"=3, "Follower"=5, "MotionProfile"=6, "MotionMagic"=7, "MotionProfileArc"=10, "Disabled"=15] ("Control Mode")
        w1687 = T13 0 items=["PercentOutput"=0, "Position"=1, "Velocity"=2, "Current"=3, "Follower"=5, "MotionProfile"=6, "MotionMagic"=7, "MotionProfileArc"=10, "Disabled"=15] ("Control Mode")
        n457 = call <vilib>:"CTRE_Phoenix_MotorControl_SetSelectedSensorPosition.vi"("error in (no error)"=w1690, "New Sensor Position"=0, "PhoenixMotorControlDevRef"=w1692) -> ("error out"=w1689:errorcluster, "PhoenixMotorControlDevRef"=w1691:T9)  [unwired: 7 in]
        n458 = Wait (ms)(milliseconds to wait=u32 20) -> ()  [unwired: 1 out]
        n459 = call <vilib>:"CTRE_Phoenix_MotorControl_Set.vi"("error in (no error)"=w1684, "Output"=0.0, "Control Mode"=w1682, "PhoenixMotorControlDevRef"=w1685) -> ("error out"=w1678:errorcluster, "PhoenixMotorControlDevRef"=w1679:T9)  [unwired: 6 in]
        n460 = call <vilib>:"CTRE_Phoenix_MotorControl_Set.vi"("error in (no error)"=w1689, "Output"=0.0, "Control Mode"=w1687, "PhoenixMotorControlDevRef"=w1691) -> ("error out"=w1680:errorcluster, "PhoenixMotorControlDevRef"=w1681:T9)  [unwired: 6 in]
        n461 = Greater?(x=w1695, y=u32 10) -> (0:w1693:bool)
      }
      n462 = while {
        tunnel: w1643 -> [w1666]
        tunnel: w1642 -> [w1667]
        tunnel: w1641 -> [w1671]
        tunnel: w1640 -> [w1670]
        tunnel: [w1665] -> w1639
        tunnel: [w1664] -> w1638
        tunnel: [w1663] -> w1637
        tunnel: [w1662] -> w1636
        i -> [w1676]
        stop <- w1674 stop-if-true
        w1668 = T13 0 items=["PercentOutput"=0, "Position"=1, "Velocity"=2, "Current"=3, "Follower"=5, "MotionProfile"=6, "MotionMagic"=7, "MotionProfileArc"=10, "Disabled"=15] ("Control Mode")
        w1673 = T13 1 items=["PercentOutput"=0, "Position"=1, "Velocity"=2, "Current"=3, "Follower"=5, "MotionProfile"=6, "MotionMagic"=7, "MotionProfileArc"=10, "Disabled"=15] ("Control Mode")
        n463 = Wait (ms)(milliseconds to wait=u32 20) -> ()  [unwired: 1 out]
        n464 = call <vilib>:"CTRE_Phoenix_MotorControl_Set.vi"("error in (no error)"=w1670, "Output"=0.0, "Control Mode"=w1668, "PhoenixMotorControlDevRef"=w1671) -> ("error out"=w1662:errorcluster, "PhoenixMotorControlDevRef"=w1663:T9)  [unwired: 6 in]
        n465 = call <vilib>:"CTRE_Phoenix_MotorControl_Set.vi"("error in (no error)"=w1667, "Output"=1024.0, "Control Mode"=w1673, "PhoenixMotorControlDevRef"=w1666) -> ("error out"=w1664:errorcluster, "PhoenixMotorControlDevRef"=w1665:T9)  [unwired: 6 in]
        n466 = Greater?(x=w1676, y=u32 10) -> (0:w1674:bool)
      }
      n467 = while {
        tunnel: w1639 -> [w1650]
        tunnel: w1638 -> [w1651]
        tunnel: w1637 -> [w1655]
        tunnel: w1636 -> [w1654]
        i -> [w1660]
        stop <- w1658 stop-if-true
        w1652 = T13 0 items=["PercentOutput"=0, "Position"=1, "Velocity"=2, "Current"=3, "Follower"=5, "MotionProfile"=6, "MotionMagic"=7, "MotionProfileArc"=10, "Disabled"=15] ("Control Mode")
        w1657 = T13 0 items=["PercentOutput"=0, "Position"=1, "Velocity"=2, "Current"=3, "Follower"=5, "MotionProfile"=6, "MotionMagic"=7, "MotionProfileArc"=10, "Disabled"=15] ("Control Mode")
        n468 = Wait (ms)(milliseconds to wait=u32 20) -> ()  [unwired: 1 out]
        n469 = call <vilib>:"CTRE_Phoenix_MotorControl_Set.vi"("error in (no error)"=w1654, "Output"=-0.1, "Control Mode"=w1652, "PhoenixMotorControlDevRef"=w1655) -> ()  [unwired: 6 in, 2 out]
        n470 = call <vilib>:"CTRE_Phoenix_MotorControl_Set.vi"("error in (no error)"=w1651, "Output"=0.0, "Control Mode"=w1657, "PhoenixMotorControlDevRef"=w1650) -> ()  [unwired: 6 in, 2 out]
        n471 = Greater?(x=w1660, y=u32 10) -> (0:w1658:bool)
      }
    }
  }
  n472 = Build Path(base path=path "/home/lvuser/natinst/bin/Paths", name or relative path=path "test1.bdx") -> (appended path=w8:path)
  n473 = call "Versioned Load.vi"("path"=w8) -> ("Trajectory Data"=w6:T14, "Fields"=w5:T18)  [unwired: 3 in, 6 out]
  n474 = Unbundle(w5) -> (w4:T19, "Angular Limits"=w2:T17)  [unwired: 3 out]
  n475 = Unbundle By Name(w4) -> ("Velocity (fps)"=w3:dbl)
  n476 = Unbundle(w2) -> ("Velocity (deg/s)"=w1:dbl)  [unwired: 2 out]
  n477 = for {
    tunnel: w6 -> [w1700] mode=indexing
    tunnel: w3 -> [w1698]
    tunnel: w1 -> [w1697]
    n478 = Unbundle By Name(w1700) -> ("Traj Vel Points"=w1699:T20)
    n479 = for {
      tunnel: w1699 -> [w1712] mode=indexing
      tunnel: w1698 -> [w1707]
      tunnel: w1697 -> [w1704]
      n480 = Unbundle(w1712) -> ("V"=w1708:dbl, "Omega"=w1705:dbl, "V vector"=w1711:cluster{"y":dbl, "x":dbl})
      n481 = call "Normalize Point.vi"("point in"=w1711) -> ("point out"=w1710:cluster{"x":sgl, "y":sgl})
      n482 = Divide(x=w1708, y=w1707) -> (x/y=w1709:dbl)
      n483 = Divide(x=w1705, y=w1704) -> (x/y=w1701:dbl)
      n484 = Multiply(x=w1710, y=w1709) -> (x*y=w1706:cluster{"x":dbl, "y":dbl})
      n485 = Unbundle(w1706) -> ("x"=w1703:dbl, "y"=w1702:dbl)
      n486 = call "Drive_Vi.vi"("Z"=w1701, "Y"=w1702, "X"=w1703) -> ()  [unwired: 9 in]
    }
  }
